vi "Athesim GUI.vi"() -> ()   [LabVIEW 2021]
uses:
  <vilib>/DAQmx/write.llb/DAQmx Write (Digital Bool 1Line 1Point).vi
  <vilib>/DAQmx/write.llb/DAQmx Write (Analog DBL 1Chan 1Samp).vi
  <vilib>/DAQmx/read.llb/DAQmx Read (Digital Bool 1Line 1Point).vi
  <vilib>/DAQmx/write.llb/DAQmx Write (Analog Wfm 1Chan NSamp).vi
  <vilib>/DAQmx/create/channels.llb/DAQmx Create Channel (DO-Digital Output).vi
  <vilib>/DAQmx/create/channels.llb/DAQmx Create Channel (DI-Digital Input).vi
  <vilib>/DAQmx/create/channels.llb/DAQmx Create Channel (AO-Voltage-Basic).vi
  <vilib>/DAQmx/miscellaneous.llb/DAQmx Fill In Error Info.vi
  <vilib>/Instr/_visa.llb/VISA Configure Serial Port (Instr).vi
  <vilib>/measure/NI_MABase.lvlib
panel:
  out "error out":errorcluster
  in  "Exposure \n(ms)":dbl=100.0
  in  "Live mode":enum32{"Static", "Strobe", "Widefield", "SIM"}(radio)=enum."Strobe"
  in  "647":bool
  in  "561":bool
  in  "488":bool
  in  "405":bool
  out "?":bool
  in  "Go live":bool
  in  "stop":bool
  in  "MG17Motor":refnum<k7>(container)
  in  "Tab Control":T1(tab)=enum."Voltages"
  in  "acquire 405":bool
  in  "405 Exp":dbl=150.0
  out "Images needed":dbl=60.0
  in  "5 phases":bool
  in  "interval /s":dbl
  in  "Timepoints":u32=5 min=1 max=1000 step=1
  in  "Steps /um":dbl
  in  "z-slices":dbl=1.0
  in  "acquire 640":bool
  in  "647 Exp":dbl=150.0
  in  "acquire 561":bool=TRUE
  in  "561 Exp":dbl=80.0
  in  "acquire 488":bool
  in  "488 Exp":dbl=150.0
  in  "Optosplit":T2(radio)=enum."rolling SIM"
  out "odd/even indicator":bool=TRUE
  out "Current voltage":dbl=0.95 format="%#_13g"
  in  "Go SIM":bool
  in  "Boolean":bool
  in  "Radio Buttons":enum32{"V1", "V2", "V3"}(radio)=enum."V3"
  in  "Debug":dbl[](array[numeric])=[0.95, 2.2, 3.45]
  out "x+y":i32=5
  in  "?":enum32{"Page 1", "Page 2", "Page 3", "Page 4"}(tab)
  in  "405 voltages":dbl[][](array[numeric])=[[1.0, 0.0, 0.0], [0.0, 0.0, 0.0], [0.0, 0.0, 4.0]]
  in  "488 voltages":dbl[][](array[numeric])=[[0.95, 2.25, 3.5], [0.951, 2.25185, 3.50055], [0.952, 2.2537, 3.5011]]
  in  "561 voltages":dbl[][](array[numeric])=[[0.95, 2.2, 3.45], [0.9506, 2.2018, 3.451], [0.9512, 2.204, 3.452]]
  in  "647 voltages":dbl[][](array[numeric])=[[0.95, 2.25, 3.5], [0.950655, 2.25185, 3.50055], [0.95131, 2.2537, 3.5011]]
  in  "?":enum32{"Page 1", "Page 2", "Page 3", "Page 4"}(tab)
  in  "405 voltages 2":dbl[][](array[numeric])=[[1.0, 0.0, 0.0], [0.0, 0.0, 0.0], [0.0, 0.0, 4.0]]
  in  "488 voltages 2":dbl[][](array[numeric])=[[0.96, 2.2, 3.5], [0.97, 2.2045, 3.51], [0.975, 2.209, 3.52]]
  in  "561 voltages 2":dbl[][](array[numeric])=[[0.85, 1.91, 3.2], [0.85065, 1.91064, 3.204], [0.85013, 1.91128, 3.208]]
  in  "647 voltages 2":dbl[][](array[numeric])=[[0.96, 2.2, 3.5], [0.97, 2.2035, 3.5085], [0.975, 2.2045, 3.5118]]
  in  "488 channel":refnum<visa-resource-name>="COM6"
  in  "ASI stage channel":refnum<visa-resource-name>="COM3"
  in  "physical channels":tag="Dev1/ao0"
  in  "expose any":tag="Dev1/port0/line5"
  in  "405 shutter":tag="Dev1/port0/line8"
  in  "Busy in":tag="Dev1/port0/line3"
  in  "Exposure out":tag="Dev1/port0/line2"
  in  "488 power":dbl(slide)=2.5974025974025974 min=0.0 max=100.0 step=0.05 scale=0.0..100.0
  in  "561 power":dbl(slide)=2.5974025974025974 min=0.0 max=100.0 step=0.05 scale=0.0..100.0
  in  "647 Power":ext(slide)=2.1 scale=0.0..100.0
  in  "488 shutter":tag="Dev1/port0/line1"
  in  "561 shutter":tag="Dev1/port0/line0"
  in  "647 channel":refnum<visa-resource-name>="COM5"
  in  "Tab Control 2":T3(tab)=enum."Page 5"
  out "Initialisation error":errorcluster
  out "stage error":errorcluster
  out "Camera/galvo error":errorcluster
  out "Laser error":errorcluster
  out "optosplit stage error":errorcluster
  out "resulting string":string="movrel z=0.000000 \r\n"
  out "resulting string 2":string="movrel z=-0.000000 \r\n"
  in  "short delay":dbl=5.0
  in  "long delay":dbl=55.0
  in  "Delay time":u32=60
  # "LIVE!"
  # "Channel"
  # "o"
  # "o"
  # "o"
  # "-60"
  # "0"
  # "60"
  # "0"
  # "2p/3"
  # "4p/3"
  # "o"
  # "o"
  # "o"
  # "-60"
  # "0"
  # "60"
  # "o"
  # "o"
  # "o"
  # "-60"
  # "0"
  # "60"
  # "o"
  # "o"
  # "o"
  # "-60"
  # "0"
  # "60"
  # "o"
  # "o"
  # "o"
  # "-60"
  # "0"
  # "60"
  # "0"
  # "3p/5"
  # "5p/5"
  # "7p/5"
  # "9p/5"
  # "o"
  # "o"
  # "o"
  # "-60"
  # "0"
  # "60"
  # "0"
  # "3p/5"
  # "5p/5"
  # "7p/5"
  # "9p/5"
  # "o"
  # "o"
  # "o"
  # "-60"
  # "0"
  # "60"
  # "0"
  # "3p/5"
  # "5p/5"
  # "7p/5"
  # "9p/5"
  # "o"
  # "o"
  # "o"
  # "-60"
  # "0"
  # "60"
  # "0"
  # "3p/5"
  # "5p/5"
  # "7p/5"
  # "9p/5"
  # "Hardware lines"
  # "Camera lines"
  # "Laser control"
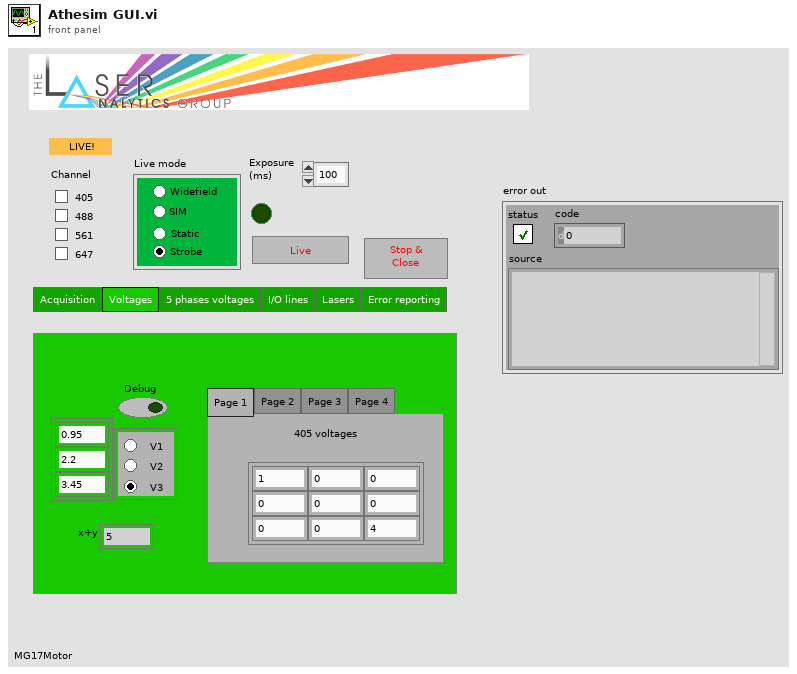
[diagram p1: front panel]
types:
  T1 = enum32{"Acquisition", "Voltages", "5 phases voltages", "I/O lines", "Lasers", "Error reporting"}
  T2 = enum32{"sequential", "optosplit", "fast sequence", "rolling SIM"}
  T3 = enum32{"Page 1", "Page 2", "Page 3", "Page 4", "Page 5"}
  T4 = enum8{"Enabled", "Disabled", "Disabled and Grayed Out"}
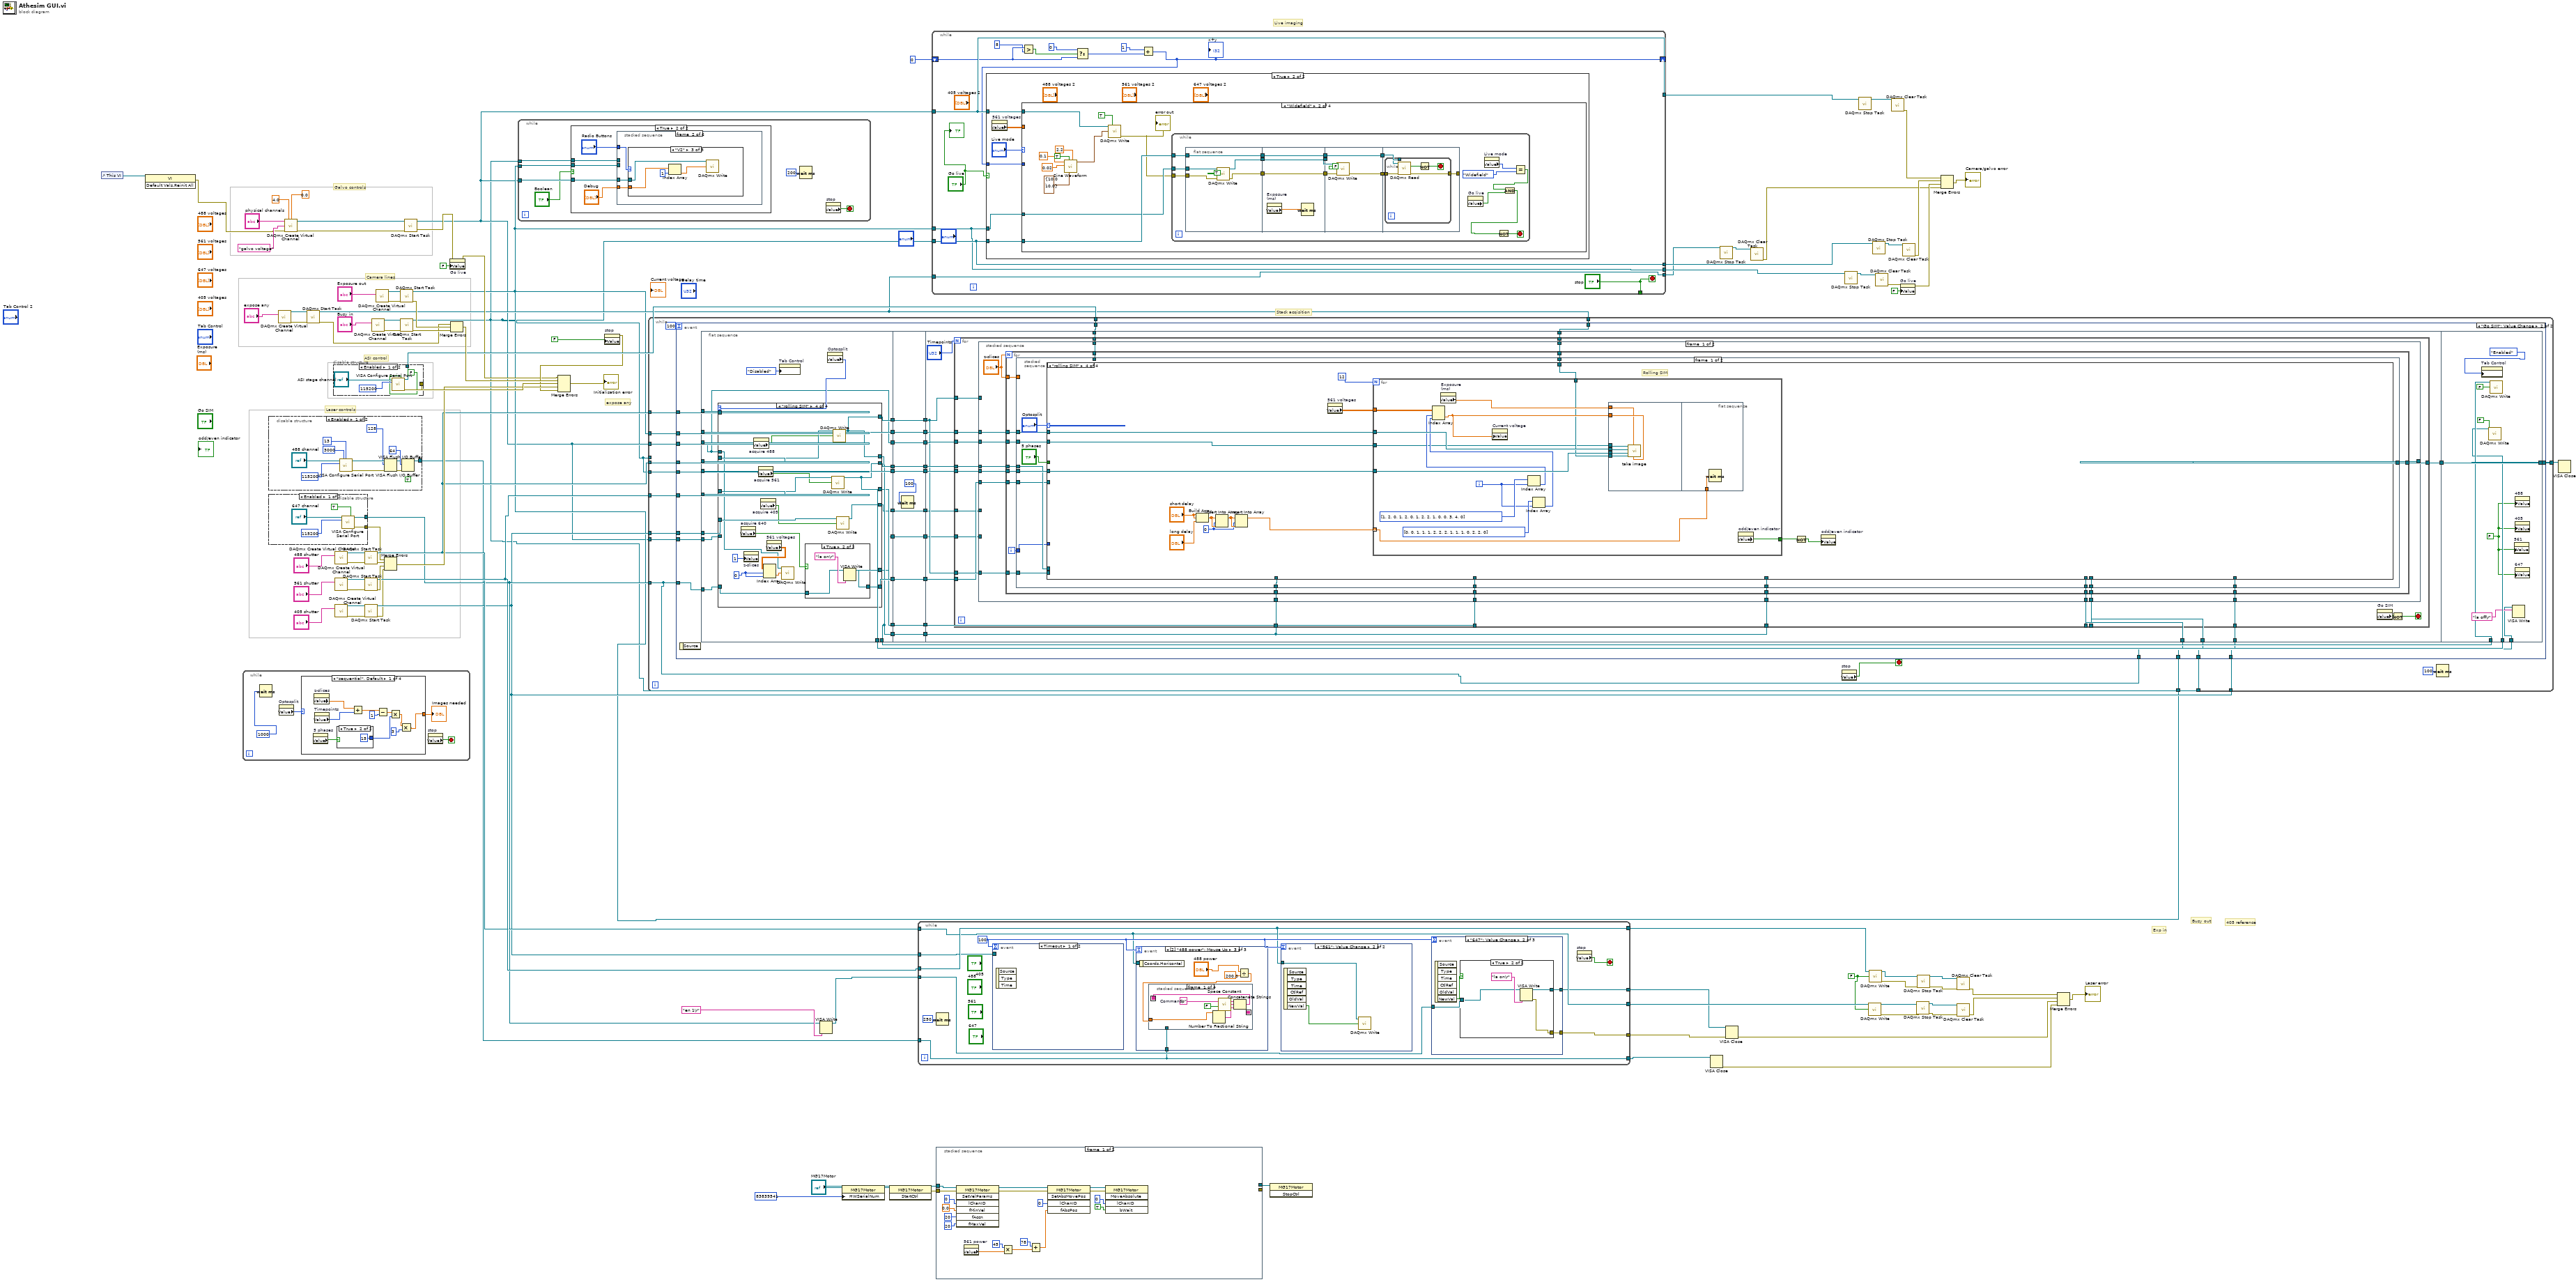
[diagram p0: block diagram]
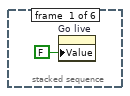
[diagram p4: hidden frame]
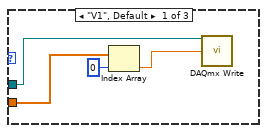
[diagram p5: hidden frame]
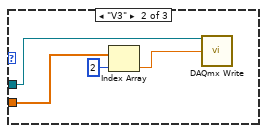
[diagram p6: hidden frame]
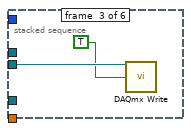
[diagram p7: hidden frame]
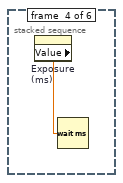
[diagram p8: hidden frame]
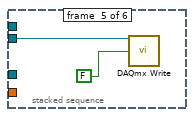
[diagram p9: hidden frame]
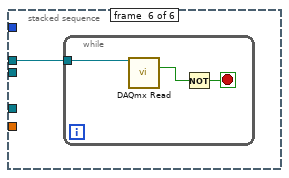
[diagram p10: hidden frame]
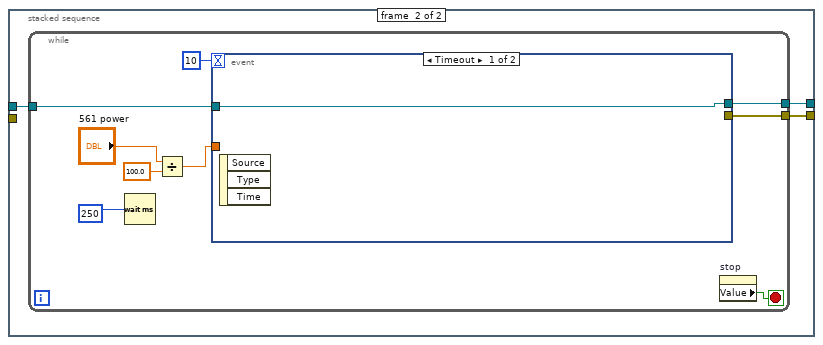
[diagram p11: hidden frame]
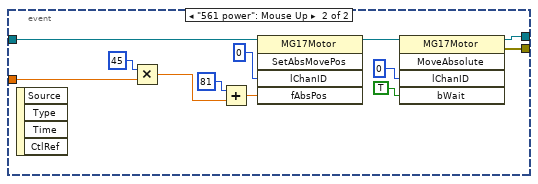
[diagram p12: hidden frame]
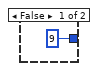
[diagram p14: hidden frame]
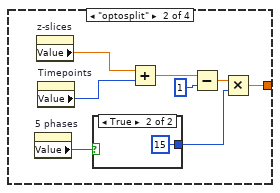
[diagram p15: hidden frame]
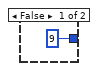
[diagram p16: hidden frame]
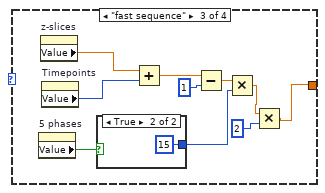
[diagram p17: hidden frame]
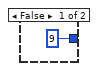
[diagram p18: hidden frame]
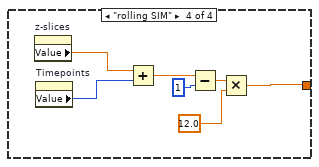
[diagram p19: hidden frame]
diagram:
  w63 = FALSE
  # "expose any"
  # "Busy out"
  # "Exp in"
  # "405 reference"
  # "Stack acqisition"
  # "Live imaging"
  # "Laser controls"
  # "ASI control"
  # "Camera lines"
  # "Galvo controls"
  n1 = control-ref of="This VI"() -> (w2:refnum<vi>)
  n2 = invoke class="VI" method="Default Vals.Reinit All"(reference=w2) -> (error out=w1:errorcluster)  [unwired: 2 in, 2 out]
  n3 = while {
    stop <- w99 stop-if-true
    n4 = Wait (ms)(milliseconds to wait=1000) -> ()  [unwired: 1 out]
    n5 = property on="Optosplit" class="RadioBtnsControl (strict)"() -> ("Value"=w98:T2)  [unwired: 2 in, 2 out]
    n6 = case shown="\"sequential\", Default" w98 {
      tunnel: [w101 w118 w123 w136] -> w100
      frame "sequential", Default {
        n7 = property on="5 phases" class="Bool (strict)"() -> ("Value"=w110:bool)  [unwired: 2 in, 2 out]
        n8 = property on="z-slices" class="DigNum (strict)"() -> ("Value"=w108:dbl)  [unwired: 2 in, 2 out]
        n9 = property on="Timepoints" class="DigNum (strict)"() -> ("Value"=w107:u32)  [unwired: 2 in, 2 out]
        n10 = case shown="True" w110 {
          tunnel: [9 15] -> w109
          frame False {
          }
          frame True {
          }
        }
        n11 = Add(x=w108, y=w107) -> (x+y=w105:dbl)
        n12 = Subtract(x=w105, y=1) -> (x-y=w104:dbl)
        n13 = Multiply(x=w104, y=w109) -> (x*y=w103:dbl)
        n14 = Multiply(x=w103, y=3) -> (x*y=w101:dbl)
      }
      frame "optosplit" {
        n15 = property on="5 phases" class="Bool (strict)"() -> ("Value"=w120:bool)  [unwired: 2 in, 2 out]
        n16 = property on="z-slices" class="DigNum (strict)"() -> ("Value"=w117:dbl)  [unwired: 2 in, 2 out]
        n17 = property on="Timepoints" class="DigNum (strict)"() -> ("Value"=w116:u32)  [unwired: 2 in, 2 out]
        n18 = case shown="True" w120 {
          tunnel: [9 15] -> w119
          frame False {
          }
          frame True {
          }
        }
        n19 = Add(x=w117, y=w116) -> (x+y=w114:dbl)
        n20 = Subtract(x=w114, y=1) -> (x-y=w113:dbl)
        n21 = Multiply(x=w113, y=w119) -> (x*y=w118:dbl)
      }
      frame "fast sequence" {
        n22 = property on="5 phases" class="Bool (strict)"() -> ("Value"=w132:bool)  [unwired: 2 in, 2 out]
        n23 = property on="z-slices" class="DigNum (strict)"() -> ("Value"=w130:dbl)  [unwired: 2 in, 2 out]
        n24 = property on="Timepoints" class="DigNum (strict)"() -> ("Value"=w129:u32)  [unwired: 2 in, 2 out]
        n25 = case shown="True" w132 {
          tunnel: [9 15] -> w131
          frame False {
          }
          frame True {
          }
        }
        n26 = Add(x=w130, y=w129) -> (x+y=w127:dbl)
        n27 = Subtract(x=w127, y=1) -> (x-y=w126:dbl)
        n28 = Multiply(x=w126, y=w131) -> (x*y=w125:dbl)
        n29 = Multiply(x=w125, y=2) -> (x*y=w123:dbl)
      }
      frame "rolling SIM" {
        n30 = property on="z-slices" class="DigNum (strict)"() -> ("Value"=w141:dbl)  [unwired: 2 in, 2 out]
        n31 = property on="Timepoints" class="DigNum (strict)"() -> ("Value"=w140:u32)  [unwired: 2 in, 2 out]
        n32 = Add(x=w141, y=w140) -> (x+y=w138:dbl)
        n33 = Subtract(x=w138, y=1) -> (x-y=w137:dbl)
        n34 = Multiply(x=w137, y=12.0) -> (x*y=w136:dbl)
      }
    }
    "Images needed" <- w100
    n35 = property on="stop" class="Bool (strict)"() -> ("Value"=w99:bool)  [unwired: 2 in, 2 out]
  }
  n36 = disable-structure shown="Enabled" {
    disable-tunnel: [w142 _] -> w6
    frame Enabled {
      (unwired) TRUE ("Enable Termination\nChar (T)")
      n37 = call-poly "VISA Configure Serial Port"("VISA resource name"="488 channel", "timeout (10sec)"=u32 3000, "termination char\n(0xA = '\\n' = LF)"=u8 13 ("termination char\n(0xA = '\\n' = LF)"), "baud rate (9600)"=u32 115200) -> ("VISA resource name out"=w152:refnum<visa-resource-name>, "error out"=w151:errorcluster)  [unwired: 5 in, 5 out]
      n38 = VISA Flush I/O Buffer(VISA resource name=w152, mask (16)=u16 128, error in (no error)=w151) -> (VISA resource name out=w148:refnum<visa-resource-name>, error out=w147:errorcluster)
      n39 = VISA Flush I/O Buffer(VISA resource name=w148, mask (16)=u16 64, error in (no error)=w147) -> (VISA resource name out=w142:refnum<visa-resource-name>)  [unwired: 1 out]
    }
    frame Disabled {
    }
  }
  n40 = disable-structure shown="Enabled" {
    disable-tunnel: [w154 _] -> w33
    disable-tunnel: [w153 _] -> w35
    frame Enabled {
      n41 = call-poly "VISA Configure Serial Port"("VISA resource name"="647 channel", "Enable Termination\nChar (T)"=TRUE ("Enable Termination\nChar (T)"), "baud rate (9600)"=u32 115200) -> ("VISA resource name out"=w154:refnum<visa-resource-name>, "error out"=w153:errorcluster)  [unwired: 11 in]
    }
    frame Disabled {
    }
  }
  n42 = call-poly <vilib>:"DAQmx Create Virtual Channel.vi"("lines"="expose any") -> ("task out"=w19:refnum<k21>, "error out"=w18:errorcluster)  [unwired: 13 in]
  n43 = call-poly <vilib>:"DAQmx Create Virtual Channel.vi"("maximum value"=4.0, "minimum value"=0.0, "physical channels"="physical channels", "name to assign"="galvo voltage", "error in"=w1) -> ("task out"=w12:refnum<k21>, "error out"=w11:errorcluster)  [unwired: 9 in]
  n44 = call <vilib>:"DAQmx Start Task.vi"("task/channels in"=w19, "error in"=w18) -> ("task out"=w16:refnum<k21>, "error out"=w17:errorcluster)  [unwired: 12 in]
  n45 = disable-structure shown="Enabled" {
    disable-tunnel: [w160 _] -> w80
    disable-tunnel: [w159 _] -> w51
    frame Enabled {
      n46 = call-poly "VISA Configure Serial Port"("VISA resource name"="ASI stage channel", "Enable Termination\nChar (T)"=FALSE, "baud rate (9600)"=u32 115200) -> ("VISA resource name out"=w159:refnum<visa-resource-name>, "error out"=w160:errorcluster)  [unwired: 11 in]
    }
    frame Disabled {
    }
  }
  n47 = call-poly <vilib>:"DAQmx Create Virtual Channel.vi"("lines"="488 shutter") -> ("task out"=w91:refnum<k21>, "error out"=w92:errorcluster)  [unwired: 13 in]
  n48 = call-poly <vilib>:"DAQmx Create Virtual Channel.vi"("lines"="561 shutter") -> ("task out"=w89:refnum<k21>, "error out"=w90:errorcluster)  [unwired: 13 in]
  n49 = call-poly <vilib>:"DAQmx Create Virtual Channel.vi"("lines"="405 shutter") -> ("task out"=w45:refnum<k21>, "error out"=w46:errorcluster)  [unwired: 13 in]
  n50 = call <vilib>:"DAQmx Start Task.vi"("task/channels in"=w91, "error in"=w92) -> ("task out"=w75:refnum<k21>, "error out"=w84:errorcluster)  [unwired: 12 in]
  n51 = call <vilib>:"DAQmx Start Task.vi"("task/channels in"=w89, "error in"=w90) -> ("task out"=w76:refnum<k21>, "error out"=w83:errorcluster)  [unwired: 12 in]
  n52 = call <vilib>:"DAQmx Start Task.vi"("task/channels in"=w45, "error in"=w46) -> ("task out"=w31:refnum<k21>, "error out"=w7:errorcluster)  [unwired: 12 in]
  n53 = call-poly <vilib>:"DAQmx Create Virtual Channel.vi"("lines"="Busy in") -> ("task out"=w93:refnum<k21>, "error out"=w94:errorcluster)  [unwired: 13 in]
  n54 = call-poly <vilib>:"DAQmx Create Virtual Channel.vi"("lines"="Exposure out") -> ("task out"=w96:refnum<k21>, "error out"=w95:errorcluster)  [unwired: 13 in]
  n55 = Merge Errors(w35, w84, w83, w7) -> (w78:errorcluster)
  n56 = call <vilib>:"DAQmx Start Task.vi"("task/channels in"=w96, "error in"=w95) -> ("task out"=w9:refnum<k21>, "error out"=w82:errorcluster)  [unwired: 12 in]
  n57 = call <vilib>:"DAQmx Start Task.vi"("task/channels in"=w93, "error in"=w94) -> ("task out"=w3:refnum<k21>, "error out"=w81:errorcluster)  [unwired: 12 in]
  n58 = call <vilib>:"DAQmx Start Task.vi"("task/channels in"=w12, "error in"=w11) -> ("task out"=w8:refnum<k21>, "error out"=w29:errorcluster)  [unwired: 12 in]
  n59 = property on="Go live" class="Bool (strict)"(error in=w29, "Value"=FALSE) -> (error out=w28:errorcluster)  [unwired: 1 in, 1 out]
  n60 = Merge Errors(w17, w82, w81) -> (w79:errorcluster)
  n61 = while {
    tunnel: w9 -> [w167]
    tunnel: w3 -> [w166]
    tunnel: w8 -> [w165]
    stop <- w168 stop-if-true
    n62 = case shown="True" "Boolean" {
      tunnel: w167 -> [_ w173]
      tunnel: w166 -> [_ w172]
      tunnel: w165 -> [_ w171]
      frame False {
      }
      frame True {
        n63 = stacked-sequence {
          tunnel: w173 -> [_ _ w191 _ w193 _]
          tunnel: w172 -> [_ _ _ _ _ w195]
          tunnel: "Radio Buttons" -> [_ w177 _ _ _ _]
          tunnel: "Debug" -> [_ w176 _ _ _ _]
          tunnel: w171 -> [_ w175 _ _ _ _]
          frame #0 {
            n64 = property on="Go live" class="Bool (strict)"("Value"=FALSE ("Go live")) -> ()  [unwired: 2 in, 2 out]
          }
          frame #1 {
            n65 = case shown="\"V2\"" w177 {
              tunnel: w176 -> [w180 w184 w188]
              tunnel: w175 -> [w181 w185 w189]
              frame "V1", Default {
                n66 = Index Array(array=w180, index=0) -> (element=w179:dbl)
                n67 = call-poly <vilib>:"DAQmx Write.vi"("task/channels in"=w181, "data"=w179) -> ()  [unwired: 11 in, 3 out]
              }
              frame "V3" {
                n68 = Index Array(array=w184, index=2) -> (element=w183:dbl)
                n69 = call-poly <vilib>:"DAQmx Write.vi"("task/channels in"=w185, "data"=w183) -> ()  [unwired: 11 in, 3 out]
              }
              frame "V2" {
                n70 = Index Array(array=w188, index=1) -> (element=w187:dbl)
                n71 = call-poly <vilib>:"DAQmx Write.vi"("task/channels in"=w189, "data"=w187) -> ()  [unwired: 11 in, 3 out]
              }
            }
          }
          frame #2 {
            n72 = call-poly <vilib>:"DAQmx Write.vi"("task/channels in"=w191, "data"=TRUE) -> ()  [unwired: 11 in, 3 out]
          }
          frame #3 {
            n73 = property on="Exposure \n(ms)" class="DigNum (strict)"() -> ("Value"=w192:dbl)  [unwired: 2 in, 2 out]
            n74 = Wait (ms)(milliseconds to wait=w192) -> ()  [unwired: 1 out]
          }
          frame #4 {
            n75 = call-poly <vilib>:"DAQmx Write.vi"("task/channels in"=w193, "data"=FALSE) -> ()  [unwired: 11 in, 3 out]
          }
          frame #5 {
            n76 = while {
              tunnel: w195 -> [w196]
              stop <- w198 stop-if-true
              n77 = call-poly <vilib>:"DAQmx Read.vi"("task/channels in"=w196) -> ("data"=w197:bool)  [unwired: 12 in, 2 out]
              n78 = Not(x=w197) -> (.not. x?=w198:bool)
            }
          }
        }
      }
    }
    n79 = Wait (ms)(milliseconds to wait=u32 200) -> ()  [unwired: 1 out]
    n80 = property on="stop" class="Bool (strict)"() -> ("Value"=w168:bool)  [unwired: 2 in, 2 out]
  }
  n81 = property on="stop" class="Bool (strict)"("Value"=FALSE) -> (error out=w48:errorcluster)  [unwired: 2 in, 1 out]
  n82 = Merge Errors(w28, w79, w80, w78, w48) -> (→"Initialisation error":errorcluster)
  n83 = while {
    tunnel: w9 -> [w215]
    tunnel: w3 -> [w214]
    tunnel: w8 -> [w213]
    tunnel: w75 -> [w212]
    tunnel: w76 -> [w211]
    tunnel: w75 -> [w210]
    tunnel: w51 -> [w208]
    tunnel: [w207] -> w50
    tunnel: w3 -> [_]
    tunnel: w33 -> [w205]
    tunnel: w31 -> [w206]
    tunnel: w31 -> [w204]
    tunnel: w9 -> [w203]
    tunnel: w3 -> [w202]
    tunnel: w8 -> [w201]
    tunnel: w16 -> [w200]
    stop <- w209 stop-if-true
    n84 = event shown="[1] \"Go SIM\": Value Change" {
      selector: _ -> [_ _]
      dyn-events: _ -> [_ _]
      timeout: 100 -> [_ _]
      tunnel: w215 -> [_ w256]
      tunnel: w214 -> [_ w255]
      tunnel: w213 -> [_ w254]
      tunnel: w212 -> [_ w253]
      tunnel: w211 -> [_ w252]
      tunnel: w210 -> [_ w251]
      tunnel: w208 -> [w217 w250]
      tunnel: [w217 w249] -> w207
      tunnel: w205 -> [_ w245]
      tunnel: w206 -> [_ w244]
      tunnel: w205 -> [_ w243]
      tunnel: w204 -> [_ w242]
      tunnel: w203 -> [_ w241]
      tunnel: w202 -> [_ w240]
      tunnel: w201 -> [_ w239]
      tunnel: w200 -> [_ w218]
      event Timeout {
        n85 = event-data() -> ()  [unwired: 1 in, 3 out]
      }
      event "Go SIM": Value Change {
        n86 = event-data() -> ()  [unwired: 1 in, 1 out]
        n87 = flat-sequence {
          tunnel: [w274] -> w238
          tunnel: w256 -> [w274]
          tunnel: [w273] -> w236
          tunnel: w255 -> [w273]
          tunnel: [w258] -> w234
          tunnel: w254 -> [w258]
          tunnel: w253 -> [w271]
          tunnel: w252 -> [w270]
          tunnel: w251 -> [w269]
          tunnel: [w268] -> w232
          tunnel: [w267] -> w230
          tunnel: [w263] -> w246
          tunnel: [w262] -> w247
          tunnel: w245 -> [w266]
          tunnel: w244 -> [w265]
          tunnel: [w264] -> w228
          tunnel: [w263] -> w226
          tunnel: [w262] -> w224
          tunnel: w239 -> [w261]
          tunnel: [w260] -> w221
          tunnel: [w259] -> w219
          tunnel: w238 -> [w364]
          tunnel: [w364] -> w237
          tunnel: w236 -> [w363]
          tunnel: [w363] -> w235
          tunnel: w234 -> [w362]
          tunnel: [w362] -> w233
          tunnel: w232 -> [w361]
          tunnel: [w361] -> w231
          tunnel: w230 -> [w360]
          tunnel: [w360] -> w229
          tunnel: w228 -> [w359]
          tunnel: [w359] -> w227
          tunnel: w226 -> [w358]
          tunnel: [w358] -> w225
          tunnel: w224 -> [w357]
          tunnel: [w357] -> w223
          tunnel: [w355] -> w222
          tunnel: w221 -> [w355]
          tunnel: [w354] -> w220
          tunnel: w219 -> [w354]
          tunnel: w237 -> [w381]
          tunnel: w235 -> [w380]
          tunnel: w233 -> [w379]
          tunnel: w231 -> [w378]
          tunnel: w229 -> [w369]
          tunnel: w250 -> [w377]
          tunnel: [w376] -> w248
          tunnel: w227 -> [w375]
          tunnel: w225 -> [w373]
          tunnel: w223 -> [w374]
          tunnel: w242 -> [w372]
          tunnel: w241 -> [w371]
          tunnel: w240 -> [w370]
          tunnel: w222 -> [w368]
          tunnel: w220 -> [w367]
          tunnel: w218 -> [w366]
          tunnel: [w1176] -> w249
          tunnel: w248 -> [w1176]
          tunnel: w247 -> [w1172]
          tunnel: w246 -> [w1173]
          tunnel: w243 -> [w1170]
          frame #0 {
            n88 = property on="Tab Control" class="TabCtl (strict)"("DisabledEnum"=T4."Disabled" ("Disabled")) -> ()  [unwired: 2 in, 2 out]
            n89 = property on="Optosplit" class="RadioBtnsControl (strict)"() -> ("Value"=w272:T2)  [unwired: 2 in, 2 out]
            n90 = case shown="\"rolling SIM\"" w272 {
              tunnel: w271 -> [_ _ _ _]
              tunnel: w270 -> [w285 w307 w326 w345]
              tunnel: w269 -> [w286 w308 w328 w347]
              tunnel: [w284 w306 w325 w344] -> w268
              tunnel: [w283 w305 w327 w346] -> w267
              tunnel: [w284 w306 w325 w344] -> w262
              tunnel: [w283 w305 w327 w346] -> w263
              tunnel: w266 -> [w278 w300 w323 w343]
              tunnel: w265 -> [w281 w303 w321 w342]
              tunnel: [w275 w297 w319 w340] -> w264
              tunnel: [w279 w301 w320 w341] -> w260
              tunnel: w261 -> [w276 w299 _ _]
              tunnel: [w275 w297 w319 w340] -> w259
              tunnel: w258 -> [_ _ _ w331]
              frame "sequential", Default {
                n91 = property on="odd/even indicator" class="Bool (strict)"() -> ("Value"=w277:bool)  [unwired: 2 in, 2 out]
                n92 = case shown="True" w277 {
                  tunnel: w276 -> [w292 w296]
                  frame False {
                    w290 = 2
                    n93 = property on="647 voltages" class="Arr (strict)"() -> ("Value"=w291:dbl[][])  [unwired: 2 in, 2 out]
                    n94 = Index Array(array=w291, index (row)=w290, index (col)=w290) -> (element=w289:dbl)
                    n95 = call-poly <vilib>:"DAQmx Write.vi"("task/channels in"=w292, "data"=w289) -> ()  [unwired: 11 in, 3 out]
                  }
                  frame True {
                    w294 = 0
                    n96 = property on="561 voltages" class="Arr (strict)"() -> ("Value"=w295:dbl[][])  [unwired: 2 in, 2 out]
                    n97 = Index Array(array=w295, index (row)=w294, index (col)=w294) -> (element=w293:dbl)
                    n98 = call-poly <vilib>:"DAQmx Write.vi"("task/channels in"=w296, "data"=w293) -> ()  [unwired: 11 in, 3 out]
                  }
                }
                n99 = call-poly <vilib>:"DAQmx Write.vi"("task/channels in"=w281, "data"=FALSE) -> ("task out"=w279:refnum<k21>)  [unwired: 11 in, 2 out]
                n100 = call-poly <vilib>:"DAQmx Write.vi"("task/channels in"=w285, "data"=FALSE) -> ("task out"=w284:refnum<k21>)  [unwired: 11 in, 2 out]
                n101 = call-poly <vilib>:"DAQmx Write.vi"("task/channels in"=w286, "data"=FALSE) -> ("task out"=w283:refnum<k21>)  [unwired: 11 in, 2 out]
                n102 = VISA Write(VISA resource name=w278, write buffer="la off\r" ("format string")) -> (VISA resource name out=w275:refnum<visa-resource-name>)  [unwired: 1 in, 2 out]
              }
              frame "fast sequence" {
                n103 = property on="odd/even indicator" class="Bool (strict)"() -> ("Value"=w298:bool)  [unwired: 2 in, 2 out]
                n104 = case shown="True" w298 {
                  tunnel: w299 -> [w314 w318]
                  frame False {
                    w312 = 2
                    n105 = property on="647 voltages" class="Arr (strict)"() -> ("Value"=w313:dbl[][])  [unwired: 2 in, 2 out]
                    n106 = Index Array(array=w313, index (row)=w312, index (col)=w312) -> (element=w311:dbl)
                    n107 = call-poly <vilib>:"DAQmx Write.vi"("task/channels in"=w314, "data"=w311) -> ()  [unwired: 11 in, 3 out]
                  }
                  frame True {
                    w316 = 0
                    n108 = property on="647 voltages" class="Arr (strict)"() -> ("Value"=w317:dbl[][])  [unwired: 2 in, 2 out]
                    n109 = Index Array(array=w317, index (row)=w316, index (col)=w316) -> (element=w315:dbl)
                    n110 = call-poly <vilib>:"DAQmx Write.vi"("task/channels in"=w318, "data"=w315) -> ()  [unwired: 11 in, 3 out]
                  }
                }
                n111 = call-poly <vilib>:"DAQmx Write.vi"("task/channels in"=w303, "data"=FALSE) -> ("task out"=w301:refnum<k21>)  [unwired: 11 in, 2 out]
                n112 = call-poly <vilib>:"DAQmx Write.vi"("task/channels in"=w307, "data"=FALSE) -> ("task out"=w306:refnum<k21>)  [unwired: 11 in, 2 out]
                n113 = call-poly <vilib>:"DAQmx Write.vi"("task/channels in"=w308, "data"=FALSE) -> ("task out"=w305:refnum<k21>)  [unwired: 11 in, 2 out]
                n114 = VISA Write(VISA resource name=w300, write buffer="la off\r" ("format string")) -> (VISA resource name out=w297:refnum<visa-resource-name>)  [unwired: 1 in, 2 out]
              }
              frame "optosplit" {
                n115 = call-poly <vilib>:"DAQmx Write.vi"("task/channels in"=w326, "data"=TRUE) -> ("task out"=w325:refnum<k21>)  [unwired: 11 in, 2 out]
                n116 = call-poly <vilib>:"DAQmx Write.vi"("task/channels in"=w328, "data"=TRUE) -> ("task out"=w327:refnum<k21>)  [unwired: 11 in, 2 out]
                n117 = call-poly <vilib>:"DAQmx Write.vi"("task/channels in"=w321, "data"=TRUE) -> ("task out"=w320:refnum<k21>)  [unwired: 11 in, 2 out]
                n118 = VISA Write(VISA resource name=w323, write buffer="la on\r" ("format string")) -> (VISA resource name out=w319:refnum<visa-resource-name>)  [unwired: 1 in, 2 out]
              }
              frame "rolling SIM" {
                w336 = 0
                n119 = property on="acquire 640" class="Bool (strict)"() -> ("Value"=w332:bool)  [unwired: 2 in, 2 out]
                n120 = property on="z-slices" class="DigNum (strict)"("Value"=1) -> ()  [unwired: 2 in, 2 out]
                n121 = property on="acquire 488" class="Bool (strict)"() -> ("Value"=w335:bool)  [unwired: 2 in, 2 out]
                n122 = property on="acquire 561" class="Bool (strict)"() -> ("Value"=w334:bool)  [unwired: 2 in, 2 out]
                n123 = property on="acquire 405" class="Bool (strict)"() -> ("Value"=w333:bool)  [unwired: 2 in, 2 out]
                n124 = property on="561 voltages" class="Arr (strict)"() -> ("Value"=w337:dbl[][])  [unwired: 2 in, 2 out]
                n125 = Index Array(array=w337, index (row)=w336, index (col)=w336) -> (element=w338:dbl)
                n126 = call-poly <vilib>:"DAQmx Write.vi"("task/channels in"=w331, "data"=w338) -> ()  [unwired: 11 in, 3 out]
                n127 = case shown="True" w332 {
                  tunnel: w343 -> [w349 w352]
                  tunnel: [w348 w351] -> w340
                  frame False {
                    n128 = VISA Write(VISA resource name=w349, write buffer="la off\r" ("format string")) -> (VISA resource name out=w348:refnum<visa-resource-name>)  [unwired: 1 in, 2 out]
                  }
                  frame True {
                    n129 = VISA Write(VISA resource name=w352, write buffer="la on\r" ("format string")) -> (VISA resource name out=w351:refnum<visa-resource-name>)  [unwired: 1 in, 2 out]
                  }
                }
                n130 = call-poly <vilib>:"DAQmx Write.vi"("task/channels in"=w345, "data"=w334) -> ("task out"=w344:refnum<k21>)  [unwired: 11 in, 2 out]
                n131 = call-poly <vilib>:"DAQmx Write.vi"("task/channels in"=w347, "data"=w335) -> ("task out"=w346:refnum<k21>)  [unwired: 11 in, 2 out]
                n132 = call-poly <vilib>:"DAQmx Write.vi"("task/channels in"=w342, "data"=w333) -> ("task out"=w341:refnum<k21>)  [unwired: 11 in, 2 out]
              }
            }
          }
          frame #1 {
            n133 = Wait (ms)(milliseconds to wait=100) -> ()  [unwired: 1 out]
          }
          frame #2 {
            n134 = for {
              N: "Timepoints" -> [_]
              tunnel: w381 -> [w401]
              tunnel: w380 -> [w400]
              tunnel: w379 -> [w399]
              tunnel: w378 -> [w398]
              tunnel: w369 -> [w397]
              tunnel: w377 -> [w396]
              tunnel: [w395] -> w376
              tunnel: w375 -> [w394]
              tunnel: w374 -> [w393]
              tunnel: w373 -> [w392]
              tunnel: w373 -> [w391]
              tunnel: w372 -> [w390]
              tunnel: w371 -> [w389]
              tunnel: w370 -> [w388]
              tunnel: w369 -> [w387]
              tunnel: w368 -> [w386]
              tunnel: w367 -> [w385]
              tunnel: w366 -> [w384]
              stop <- w382 stop-if-true
              n135 = stacked-sequence {
                tunnel: w401 -> [w417 _]
                tunnel: w400 -> [w416 _]
                tunnel: w399 -> [w415 _]
                tunnel: w398 -> [w414 w1081]
                tunnel: w397 -> [w413 _]
                tunnel: w396 -> [w412 w1083]
                tunnel: [w411 _] -> w395
                tunnel: w394 -> [w410 _]
                tunnel: w393 -> [w409 _]
                tunnel: w392 -> [w408 _]
                tunnel: w391 -> [w407 _]
                tunnel: w390 -> [w406 _]
                tunnel: w389 -> [w405 _]
                tunnel: w388 -> [w404 _]
                tunnel: w387 -> [_ w1082]
                tunnel: w386 -> [_ w1080]
                tunnel: w385 -> [_ w1079]
                tunnel: w384 -> [w402 _]
                frame #0 {
                  n136 = for {
                    N: "z-slices" -> [_]
                    tunnel: w417 -> [w434]
                    tunnel: w416 -> [w433]
                    tunnel: w415 -> [w432]
                    tunnel: w414 -> [w431]
                    tunnel: w413 -> [w430]
                    tunnel: w412 -> [w429]
                    tunnel: [w428] -> w411
                    tunnel: w410 -> [w427]
                    tunnel: w409 -> [w426]
                    tunnel: w408 -> [w425]
                    tunnel: w407 -> [w424]
                    tunnel: w406 -> [w423]
                    tunnel: w405 -> [w422]
                    tunnel: w404 -> [w421]
                    tunnel: "z-slices" -> [w419]
                    tunnel: w402 -> [w418]
                    i -> [w420]
                    n137 = stacked-sequence {
                      tunnel: w434 -> [w449 _]
                      tunnel: w433 -> [w448 _]
                      tunnel: w432 -> [w447 _]
                      tunnel: w431 -> [w446 _]
                      tunnel: w430 -> [w445 _]
                      tunnel: w429 -> [_ w1051]
                      tunnel: [_ w1050] -> w428
                      tunnel: w427 -> [w443 _]
                      tunnel: w426 -> [w442 _]
                      tunnel: w425 -> [w441 _]
                      tunnel: w424 -> [w440 _]
                      tunnel: w423 -> [w439 _]
                      tunnel: w422 -> [w438 _]
                      tunnel: w421 -> [w437 _]
                      tunnel: w420 -> [w436 _]
                      tunnel: w419 -> [_ w1046]
                      tunnel: w418 -> [w435 _]
                      frame #0 {
                        n138 = case shown="\"rolling SIM\"" "Optosplit" {
                          tunnel: w449 -> [w472 w795 w924 w1021]
                          tunnel: w448 -> [w471 w794 w923 w1020]
                          tunnel: w447 -> [w454 w790 w922 w1014]
                          tunnel: w446 -> [w461 _ _ _]
                          tunnel: w445 -> [w460 _ _ _]
                          tunnel: "5 phases" -> [_ _ w921 _]
                          tunnel: w443 -> [w459 w789 _ _]
                          tunnel: w442 -> [w458 w788 _ _]
                          tunnel: w441 -> [w457 _ _ _]
                          tunnel: w440 -> [_ w783 _ _]
                          tunnel: w439 -> [w456 w782 _ _]
                          tunnel: w438 -> [w453 _ _ _]
                          tunnel: w437 -> [w452 _ _ _]
                          tunnel: w436 -> [_ _ _ _]
                          tunnel: w435 -> [w451 w781 w920 w1015]
                          frame "sequential", Default {
                            # "Without optosplit"
                            n139 = case shown="True" "acquire 640" {
                              tunnel: w472 -> [w700 w710]
                              tunnel: w471 -> [w698 w709]
                              tunnel: w454 -> [w699 w703]
                              tunnel: [w700 w707] -> w467
                              tunnel: [w699 w708] -> w468
                              tunnel: [w698 w706] -> w469
                              tunnel: w459 -> [_ w702]
                              tunnel: w451 -> [_ w701]
                              frame False {
                              }
                              frame True {
                                n140 = property on="647 voltages" class="Arr (strict)"() -> ("Value"=w704:dbl[][])  [unwired: 2 in, 2 out]
                                n141 = stacked-sequence {
                                seq-local: [_ w724 _ _] -> [_ _ w744 _]
                                seq-local: [_ w723 _ _] -> [_ _ w743 _]
                                seq-local: [_ w722 _ _] -> [_ _ w742 _]
                                seq-local: [_ w721 _ _] -> [_ _ w738 _]
                                seq-local: [_ w720 _ _] -> [_ _ w737 _]
                                tunnel: w710 -> [_ w724 _ _]
                                tunnel: w703 -> [_ w723 _ _]
                                tunnel: w709 -> [_ w722 _ _]
                                tunnel: w704 -> [_ w721 _ _]
                                tunnel: "647 Exp" -> [_ w720 _ _]
                                tunnel: [_ _ w741 _] -> w708
                                tunnel: [_ _ w740 _] -> w707
                                tunnel: [_ _ w739 _] -> w706
                                tunnel: w704 -> [_ w719 _ _]
                                tunnel: w703 -> [_ w718 _ _]
                                tunnel: w702 -> [w711 _ _ w778]
                                tunnel: w701 -> [_ _ w735 _]
                                frame #0 {
                                n142 = stacked-sequence {
                                tunnel: w711 -> [w712 _]
                                frame #0 {
                                n143 = VISA Write(VISA resource name=w712, write buffer="la on\r" ("format string")) -> ()  [unwired: 1 in, 3 out]
                                }
                                frame #1 {
                                n144 = Wait (ms)(milliseconds to wait=100) -> ()  [unwired: 1 out]
                                }
                                }
                                }
                                frame #1 {
                                n145 = property on="odd/even indicator" class="Bool (strict)"() -> ("Value"=w715:bool)  [unwired: 2 in, 2 out]
                                n146 = case shown="False" w715 {
                                tunnel: [2 0] -> w717
                                tunnel: [2 0] -> w716
                                frame False {
                                }
                                frame True {
                                }
                                }
                                n147 = flat-sequence {
                                tunnel: [w732] -> _
                                tunnel: w719 -> [w734]
                                tunnel: w718 -> [w732]
                                tunnel: [w733] -> _
                                tunnel: w717 -> [w730]
                                tunnel: w716 -> [w729]
                                frame #0 {
                                n148 = Index Array(array=w734, index (row)=w730, index (col)=w729) -> (element=w731:dbl)
                                n149 = call-poly <vilib>:"DAQmx Write.vi"("task/channels in"=w732, "data"=w731) -> ("task out"=w733:refnum<k21>)  [unwired: 11 in, 2 out]
                                }
                                }
                                }
                                frame #2 {
                                n150 = for {
                                N: 9 -> [_]
                                tunnel: w738 -> [w756]
                                tunnel: w744 -> [w753]
                                tunnel: w743 -> [w754]
                                tunnel: w742 -> [w752]
                                tunnel: w737 -> [w755]
                                tunnel: [w754] -> w741
                                tunnel: [w753] -> w740
                                tunnel: [w752] -> w739
                                tunnel: w735 -> [w745]
                                i -> [w748]
                                n151 = property on="odd/even indicator" class="Bool (strict)"() -> ("Value"=w746:bool)  [unwired: 2 in, 2 out]
                                n152 = case shown="True" w746 {
                                tunnel: [i32[] [1, 0, 2, 1, 0, 2, 1, 0, 0, 0, 1, 2, 3, 4, 0] i32[] [1, 2, 0, 1, 2, 0, 1, 2, 2, 0, 1, 2, 3, 4, 0]] -> w751
                                tunnel: [i32[] [2, 2, 1, 1, 1, 0, 0, 0, 0, 2, 2, 2, 2, 2, 0] i32[] [0, 0, 1, 1, 1, 2, 2, 2, 2, 2, 2, 2, 2, 2, 0]] -> w750
                                frame False {
                                }
                                frame True {
                                }
                                }
                                n153 = Index Array(array=w751, index=w748) -> (element=w749:i32)
                                n154 = flat-sequence {
                                tunnel: w756 -> [w765]
                                tunnel: w755 -> [w769]
                                tunnel: w754 -> [w768]
                                tunnel: w753 -> [w767]
                                tunnel: w752 -> [w766]
                                tunnel: w747 -> [w763]
                                tunnel: w749 -> [w762]
                                tunnel: w745 -> [w761]
                                frame #0 {
                                n155 = Index Array(array=w765, index (row)=w762, index (col)=w763) -> (element=w764:dbl)
                                n156 = call "take image.vi"("Voltage"=w764, "Exposure time"=w769, "expose any"=w761, "Busy out"=w766, "Exp In"=w767, "Galvo"=w768) -> ()  [unwired: 6 in]
                                }
                                frame #1 {
                                n157 = property on="Delay time" class="DigNum (strict)"() -> ("Value"=w770:u32)  [unwired: 2 in, 2 out]
                                n158 = Wait (ms)(milliseconds to wait=w770) -> ()  [unwired: 1 out]
                                }
                                }
                                n159 = Index Array(array=w750, index=w748) -> (element=w747:i32)
                                }
                                }
                                frame #3 {
                                n160 = property on="acquire 488" class="Bool (strict)"() -> ("Value"=w774:bool)  [unwired: 2 in, 2 out]
                                n161 = property on="acquire 405" class="Bool (strict)"() -> ("Value"=w773:bool)  [unwired: 2 in, 2 out]
                                n162 = property on="acquire 561" class="Bool (strict)"() -> ("Value"=w775:bool)  [unwired: 2 in, 2 out]
                                n163 = property on="odd/even indicator" class="Bool (strict)"() -> ("Value"=w776:bool)  [unwired: 2 in, 2 out]
                                n164 = Or(x=w775, y=w774) -> (x .or. y?=w772:bool)
                                n165 = Not(x=w776) -> (.not. x?=w777:bool)
                                n166 = Or(x=w772, y=w773) -> (x .or. y?=w771:bool)
                                n167 = case shown="True" w771 {
                                tunnel: w778 -> [_ w779]
                                frame False {
                                }
                                frame True {
                                n168 = VISA Write(VISA resource name=w779, write buffer="la off\r" ("format string")) -> ()  [unwired: 1 in, 3 out]
                                }
                                }
                                n169 = property on="odd/even indicator" class="Bool (strict)"("Value"=w777) -> ()  [unwired: 2 in, 2 out]
                                }
                                }
                              }
                            }
                            n170 = case shown="True" "acquire 561" {
                              tunnel: w469 -> [w617 w628]
                              tunnel: w468 -> [w618 w629]
                              tunnel: [w616 w626] -> w465
                              tunnel: [w618 w627] -> w464
                              tunnel: [w617 w625] -> w463
                              tunnel: w467 -> [w616 w624]
                              tunnel: w461 -> [_ _]
                              tunnel: w454 -> [_ w621]
                              tunnel: w458 -> [_ w620]
                              tunnel: w451 -> [_ w619]
                              frame False {
                              }
                              frame True {
                                n171 = property on="561 voltages" class="Arr (strict)"() -> ("Value"=w622:dbl[][])  [unwired: 2 in, 2 out]
                                n172 = stacked-sequence {
                                seq-local: [_ w639 _ _] -> [_ _ w661 _]
                                seq-local: [_ w638 _ _] -> [_ _ w660 _]
                                seq-local: [_ w637 _ _] -> [_ _ w656 _]
                                seq-local: [_ w636 _ _] -> [_ _ w654 _]
                                seq-local: [_ w635 _ _] -> [_ _ w653 _]
                                tunnel: w629 -> [_ w639 _ _]
                                tunnel: w628 -> [_ w638 _ _]
                                tunnel: w624 -> [_ w637 _ _]
                                tunnel: w622 -> [_ w636 _ _]
                                tunnel: "561 Exp" -> [_ w635 _ _]
                                tunnel: [_ _ w659 _] -> w627
                                tunnel: [_ _ w658 _] -> w626
                                tunnel: [_ _ w657 _] -> w625
                                tunnel: w622 -> [_ w633 _ _]
                                tunnel: w621 -> [_ w632 _ _]
                                tunnel: w620 -> [w631 _ _ w695]
                                tunnel: w619 -> [_ _ w652 _]
                                frame #0 {
                                n173 = call-poly <vilib>:"DAQmx Write.vi"("task/channels in"=w631, "data"=TRUE) -> ()  [unwired: 11 in, 3 out]
                                }
                                frame #1 {
                                n174 = flat-sequence {
                                tunnel: w633 -> [w643]
                                tunnel: [w642] -> w634
                                tunnel: w632 -> [w641]
                                tunnel: [w651] -> _
                                tunnel: w634 -> [w651]
                                frame #0 {
                                n175 = property on="odd/even indicator" class="Bool (strict)"() -> ("Value"=w640:bool)  [unwired: 2 in, 2 out]
                                n176 = case shown="True" w640 {
                                tunnel: [2 0] -> w646
                                tunnel: [2 0] -> w645
                                frame False {
                                }
                                frame True {
                                }
                                }
                                n177 = Index Array(array=w643, index (row)=w646, index (col)=w645) -> (element=w644:dbl)
                                n178 = call-poly <vilib>:"DAQmx Write.vi"("task/channels in"=w641, "data"=w644) -> ("task out"=w642:refnum<k21>)  [unwired: 11 in, 2 out]
                                }
                                frame #1 {
                                }
                                }
                                }
                                frame #2 {
                                n179 = for {
                                N: 9 -> [_]
                                tunnel: w654 -> [w673]
                                tunnel: w656 -> [w670]
                                tunnel: w661 -> [w671]
                                tunnel: w660 -> [w669]
                                tunnel: w653 -> [w672]
                                tunnel: [w671] -> w659
                                tunnel: [w670] -> w658
                                tunnel: [w669] -> w657
                                tunnel: w652 -> [w662]
                                i -> [w666]
                                n180 = property on="odd/even indicator" class="Bool (strict)"() -> ("Value"=w663:bool)  [unwired: 2 in, 2 out]
                                n181 = case shown="False" w663 {
                                tunnel: [i32[] [2, 2, 1, 1, 1, 0, 0, 0, 0, 2, 2, 2, 2, 2, 0] i32[] [0, 0, 1, 1, 1, 2, 2, 2, 2, 2, 2, 2, 2, 2, 0]] -> w668
                                tunnel: [i32[] [1, 0, 2, 1, 0, 2, 1, 0, 0, 0, 1, 2, 3, 4, 0] i32[] [1, 2, 0, 1, 2, 0, 1, 2, 2, 0, 1, 2, 3, 4, 0]] -> w667
                                frame False {
                                }
                                frame True {
                                }
                                }
                                n182 = flat-sequence {
                                tunnel: w673 -> [w682]
                                tunnel: w672 -> [w686]
                                tunnel: w671 -> [w685]
                                tunnel: w670 -> [w684]
                                tunnel: w669 -> [w683]
                                tunnel: w665 -> [w680]
                                tunnel: w664 -> [w679]
                                tunnel: w662 -> [w678]
                                frame #0 {
                                n183 = Index Array(array=w682, index (row)=w680, index (col)=w679) -> (element=w681:dbl)
                                n184 = call "take image.vi"("Voltage"=w681, "Exposure time"=w686, "expose any"=w678, "Busy out"=w683, "Exp In"=w684, "Galvo"=w685) -> ()  [unwired: 6 in]
                                }
                                frame #1 {
                                n185 = property on="Delay time" class="DigNum (strict)"() -> ("Value"=w687:u32)  [unwired: 2 in, 2 out]
                                n186 = Wait (ms)(milliseconds to wait=w687) -> ()  [unwired: 1 out]
                                }
                                }
                                n187 = Index Array(array=w667, index=w666) -> (element=w665:i32)
                                n188 = Index Array(array=w668, index=w666) -> (element=w664:i32)
                                }
                                }
                                frame #3 {
                                n189 = property on="acquire 488" class="Bool (strict)"() -> ("Value"=w691:bool)  [unwired: 2 in, 2 out]
                                n190 = property on="acquire 405" class="Bool (strict)"() -> ("Value"=w692:bool)  [unwired: 2 in, 2 out]
                                n191 = property on="acquire 640" class="Bool (strict)"() -> ("Value"=w690:bool)  [unwired: 2 in, 2 out]
                                n192 = Or(x=w691, y=w692) -> (x .or. y?=w689:bool)
                                n193 = Or(x=w689, y=w690) -> (x .or. y?=w688:bool)
                                n194 = case shown="False" w688 {
                                tunnel: w695 -> [_ w696]
                                frame False {
                                }
                                frame True {
                                n195 = call-poly <vilib>:"DAQmx Write.vi"("task/channels in"=w696, "data"=FALSE) -> ()  [unwired: 11 in, 3 out]
                                }
                                }
                                n196 = property on="odd/even indicator" class="Bool (strict)"() -> ("Value"=w694:bool)  [unwired: 2 in, 2 out]
                                n197 = Not(x=w694) -> (.not. x?=w693:bool)
                                n198 = property on="odd/even indicator" class="Bool (strict)"("Value"=w693) -> ()  [unwired: 2 in, 2 out]
                                }
                                }
                              }
                            }
                            n199 = case shown="True" "acquire 488" {
                              tunnel: w465 -> [w538 w544]
                              tunnel: w463 -> [w536 w548]
                              tunnel: w464 -> [w537 w549]
                              tunnel: [w538 w546] -> _
                              tunnel: [w537 w547] -> _
                              tunnel: [w536 w545] -> _
                              tunnel: w460 -> [_ _]
                              tunnel: w454 -> [_ w541]
                              tunnel: w457 -> [_ w540]
                              tunnel: w451 -> [_ w539]
                              frame False {
                              }
                              frame True {
                                n200 = property on="488 voltages" class="Arr (strict)"() -> ("Value"=w542:dbl[][])  [unwired: 2 in, 2 out]
                                n201 = stacked-sequence {
                                seq-local: [_ w558 _ _] -> [_ _ w579 _]
                                seq-local: [_ w557 _ _] -> [_ _ w578 _]
                                seq-local: [_ w556 _ _] -> [_ _ w574 _]
                                seq-local: [_ w555 _ _] -> [_ _ w572 _]
                                seq-local: [_ w554 _ _] -> [_ _ w571 _]
                                tunnel: w549 -> [_ w558 _ _]
                                tunnel: w548 -> [_ w557 _ _]
                                tunnel: w544 -> [_ w556 _ _]
                                tunnel: w542 -> [_ w555 _ _]
                                tunnel: "488 Exp" -> [_ w554 _ _]
                                tunnel: [_ _ w577 _] -> w547
                                tunnel: [_ _ w576 _] -> w546
                                tunnel: [_ _ w575 _] -> w545
                                tunnel: w542 -> [_ w553 _ _]
                                tunnel: w541 -> [_ w552 _ _]
                                tunnel: w540 -> [w550 _ _ w613]
                                tunnel: w539 -> [_ _ w570 _]
                                frame #0 {
                                n202 = call-poly <vilib>:"DAQmx Write.vi"("task/channels in"=w550, "data"=TRUE) -> ()  [unwired: 11 in, 3 out]
                                }
                                frame #1 {
                                n203 = flat-sequence {
                                tunnel: w553 -> [w565]
                                tunnel: w552 -> [w563]
                                tunnel: [w564] -> _
                                frame #0 {
                                n204 = property on="odd/even indicator" class="Bool (strict)"() -> ("Value"=w559:bool)  [unwired: 2 in, 2 out]
                                n205 = case shown="False" w559 {
                                tunnel: [2 0] -> w561
                                tunnel: [2 0] -> w560
                                frame False {
                                }
                                frame True {
                                }
                                }
                                n206 = Index Array(array=w565, index (row)=w561, index (col)=w560) -> (element=w562:dbl)
                                n207 = call-poly <vilib>:"DAQmx Write.vi"("task/channels in"=w563, "data"=w562) -> ("task out"=w564:refnum<k21>)  [unwired: 11 in, 2 out]
                                }
                                }
                                }
                                frame #2 {
                                n208 = for {
                                N: 9 -> [_]
                                tunnel: w572 -> [w591]
                                tunnel: w574 -> [w589]
                                tunnel: w579 -> [w590]
                                tunnel: w578 -> [w588]
                                tunnel: [w590] -> w577
                                tunnel: [w589] -> w576
                                tunnel: [w588] -> w575
                                tunnel: w571 -> [w587]
                                tunnel: w570 -> [w580]
                                i -> [w586]
                                n209 = property on="odd/even indicator" class="Bool (strict)"() -> ("Value"=w581:bool)  [unwired: 2 in, 2 out]
                                n210 = case shown="True" w581 {
                                tunnel: [i32[] [2, 2, 1, 1, 1, 0, 0, 0, 0, 2, 2, 2, 2, 2, 0] i32[] [0, 0, 1, 1, 1, 2, 2, 2, 2, 2, 2, 2, 2, 2, 0]] -> w582
                                tunnel: [i32[] [1, 0, 2, 1, 0, 2, 1, 0, 0, 0, 1, 2, 3, 4, 0] i32[] [1, 2, 0, 1, 2, 0, 1, 2, 2, 0, 1, 2, 3, 4, 0]] -> w583
                                frame False {
                                }
                                frame True {
                                }
                                }
                                n211 = Index Array(array=w583, index=w586) -> (element=w585:i32)
                                n212 = Index Array(array=w582, index=w586) -> (element=w584:i32)
                                n213 = flat-sequence {
                                tunnel: w591 -> [w600]
                                tunnel: w587 -> [w604]
                                tunnel: w590 -> [w603]
                                tunnel: w589 -> [w602]
                                tunnel: w588 -> [w601]
                                tunnel: w585 -> [w598]
                                tunnel: w584 -> [w597]
                                tunnel: w580 -> [w596]
                                frame #0 {
                                n214 = Index Array(array=w600, index (row)=w598, index (col)=w597) -> (element=w599:dbl)
                                n215 = call "take image.vi"("Voltage"=w599, "Exposure time"=w604, "expose any"=w596, "Busy out"=w601, "Exp In"=w602, "Galvo"=w603) -> ()  [unwired: 6 in]
                                }
                                frame #1 {
                                n216 = property on="Delay time" class="DigNum (strict)"() -> ("Value"=w605:u32)  [unwired: 2 in, 2 out]
                                n217 = Wait (ms)(milliseconds to wait=w605) -> ()  [unwired: 1 out]
                                }
                                }
                                }
                                }
                                frame #3 {
                                n218 = property on="acquire 561" class="Bool (strict)"() -> ("Value"=w609:bool)  [unwired: 2 in, 2 out]
                                n219 = property on="acquire 405" class="Bool (strict)"() -> ("Value"=w608:bool)  [unwired: 2 in, 2 out]
                                n220 = property on="acquire 640" class="Bool (strict)"() -> ("Value"=w610:bool)  [unwired: 2 in, 2 out]
                                n221 = property on="odd/even indicator" class="Bool (strict)"() -> ("Value"=w611:bool)  [unwired: 2 in, 2 out]
                                n222 = Not(x=w611) -> (.not. x?=w612:bool)
                                n223 = Or(x=w609, y=w608) -> (x .or. y?=w607:bool)
                                n224 = property on="odd/even indicator" class="Bool (strict)"("Value"=w612) -> ()  [unwired: 2 in, 2 out]
                                n225 = Or(x=w607, y=w610) -> (x .or. y?=w606:bool)
                                n226 = case shown="True" w606 {
                                tunnel: w613 -> [_ w614]
                                frame False {
                                }
                                frame True {
                                n227 = call-poly <vilib>:"DAQmx Write.vi"("task/channels in"=w614, "data"=FALSE) -> ()  [unwired: 11 in, 3 out]
                                }
                                }
                                }
                                }
                              }
                            }
                            n228 = case shown="True" "acquire 405" {
                              tunnel: w456 -> [_ w479]
                              tunnel: w454 -> [_ w477]
                              tunnel: w453 -> [_ w475]
                              tunnel: w452 -> [_ w474]
                              tunnel: w451 -> [_ w473]
                              frame False {
                              }
                              frame True {
                                n229 = property on="405 voltages" class="Arr (strict)"() -> ("Value"=w478:dbl[][])  [unwired: 2 in, 2 out]
                                n230 = stacked-sequence {
                                tunnel: w478 -> [_ w483 w498 _]
                                tunnel: w477 -> [_ w482 w497 _]
                                tunnel: [_ _ _ w533] -> _
                                tunnel: w479 -> [w480 _ _ w533]
                                tunnel: "405 Exp" -> [_ _ w496 _]
                                tunnel: w475 -> [_ _ w495 _]
                                tunnel: w474 -> [_ _ w494 _]
                                tunnel: w473 -> [_ _ w493 _]
                                frame #0 {
                                n231 = call-poly <vilib>:"DAQmx Write.vi"("task/channels in"=w480, "data"=TRUE) -> ()  [unwired: 11 in, 3 out]
                                }
                                frame #1 {
                                n232 = flat-sequence {
                                tunnel: w483 -> [w487]
                                tunnel: [w486] -> w484
                                tunnel: w482 -> [w485]
                                tunnel: [w492] -> _
                                tunnel: w484 -> [w492]
                                frame #0 {
                                n233 = Index Array(array=w487, index (row)=0, index (col)=0) -> (element=w488:dbl)
                                n234 = call-poly <vilib>:"DAQmx Write.vi"("task/channels in"=w485, "data"=w488) -> ("task out"=w486:refnum<k21>)  [unwired: 11 in, 2 out]
                                }
                                frame #1 {
                                n235 = Wait (ms)(milliseconds to wait=50) -> ()  [unwired: 1 out]
                                }
                                }
                                }
                                frame #2 {
                                n236 = for {
                                N: 9 -> [_]
                                tunnel: w498 -> [w509]
                                tunnel: w497 -> [w508]
                                tunnel: w496 -> [w507]
                                tunnel: w495 -> [w506]
                                tunnel: w494 -> [w505]
                                tunnel: w493 -> [w500]
                                i -> [w504]
                                n237 = property on="odd/even indicator" class="Bool (strict)"() -> ("Value"=w501:bool)  [unwired: 2 in, 2 out]
                                n238 = case shown="True" w501 {
                                tunnel: [i32[] [2, 2, 1, 1, 1, 0, 0, 0, 0, 2, 2, 2, 2, 2, 0] i32[] [0, 0, 1, 1, 1, 2, 2, 2, 2, 2, 2, 2, 2, 2, 0]] -> w503
                                tunnel: [i32[] [1, 0, 2, 1, 0, 2, 1, 0, 0, 0, 1, 2, 3, 4, 0] i32[] [1, 2, 0, 1, 2, 0, 1, 2, 2, 0, 1, 2, 3, 4, 0]] -> w502
                                frame False {
                                }
                                frame True {
                                }
                                }
                                n239 = flat-sequence {
                                tunnel: w511 -> [w523]
                                tunnel: w510 -> [w522]
                                tunnel: w509 -> [w521]
                                tunnel: w508 -> [w520]
                                tunnel: w507 -> [w519]
                                tunnel: w506 -> [w518]
                                tunnel: w505 -> [w517]
                                tunnel: w500 -> [w516]
                                frame #0 {
                                n240 = Index Array(array=w521, index (row)=w523, index (col)=w522) -> (element=w524:dbl)
                                n241 = call "take image.vi"("Voltage"=w524, "Exposure time"=w519, "expose any"=w516, "Busy out"=w517, "Exp In"=w518, "Galvo"=w520) -> ()  [unwired: 6 in]
                                }
                                frame #1 {
                                n242 = property on="Delay time" class="DigNum (strict)"() -> ("Value"=w525:u32)  [unwired: 2 in, 2 out]
                                n243 = Wait (ms)(milliseconds to wait=w525) -> ()  [unwired: 1 out]
                                }
                                }
                                n244 = Index Array(array=w502, index=w504) -> (element=w511:i32)
                                n245 = Index Array(array=w503, index=w504) -> (element=w510:i32)
                                }
                                }
                                frame #3 {
                                n246 = property on="acquire 561" class="Bool (strict)"() -> ("Value"=w528:bool)  [unwired: 2 in, 2 out]
                                n247 = property on="acquire 488" class="Bool (strict)"() -> ("Value"=w529:bool)  [unwired: 2 in, 2 out]
                                n248 = property on="acquire 640" class="Bool (strict)"() -> ("Value"=w527:bool)  [unwired: 2 in, 2 out]
                                n249 = Or(x=w528, y=w529) -> (x .or. y?=w530:bool)
                                n250 = property on="odd/even indicator" class="Bool (strict)"() -> ("Value"=w532:bool)  [unwired: 2 in, 2 out]
                                n251 = Or(x=w530, y=w527) -> (x .or. y?=w526:bool)
                                n252 = Not(x=w532) -> (.not. x?=w531:bool)
                                n253 = property on="odd/even indicator" class="Bool (strict)"("Value"=w531) -> ()  [unwired: 2 in, 2 out]
                                n254 = case shown="True" w526 {
                                tunnel: w533 -> [_ w534]
                                frame False {
                                }
                                frame True {
                                n255 = call-poly <vilib>:"DAQmx Write.vi"("task/channels in"=w534, "data"=FALSE) -> ()  [unwired: 11 in, 3 out]
                                }
                                }
                                }
                                }
                              }
                            }
                          }
                          frame "fast sequence" {
                            # "561"
                            # "488"
                            # "fast sequence"
                            n256 = property on="647 Exp" class="DigNum (strict)"() -> ("Value"=w784:dbl)  [unwired: 2 in, 2 out]
                            n257 = property on="647 voltages" class="Arr (strict)"() -> ("Value"=w787:dbl[][])  [unwired: 2 in, 2 out]
                            n258 = stacked-sequence {
                              seq-local: [_ w869 _ _] -> [_ _ w887 _]
                              seq-local: [_ w868 _ _] -> [_ _ w886 _]
                              seq-local: [_ w867 _ _] -> [_ _ w885 _]
                              seq-local: [_ w866 _ _] -> [_ _ w881 _]
                              seq-local: [_ w865 _ _] -> [_ _ w880 _]
                              tunnel: w795 -> [_ w869 _ _]
                              tunnel: w790 -> [_ w868 _ _]
                              tunnel: w794 -> [_ w867 _ _]
                              tunnel: w787 -> [_ w866 _ _]
                              tunnel: w784 -> [_ w865 _ _]
                              tunnel: [_ _ w884 _] -> w792
                              tunnel: [_ _ w883 _] -> w791
                              tunnel: [_ _ w882 _] -> w793
                              tunnel: w787 -> [_ w863 _ _]
                              tunnel: w790 -> [_ w862 _ _]
                              tunnel: w789 -> [w860 _ _ w918]
                              tunnel: w783 -> [w858 _ _ w916]
                              tunnel: w781 -> [_ _ w878 _]
                              frame #0 {
                                n259 = VISA Write(VISA resource name=w860, write buffer="la on\r" ("format string")) -> ()  [unwired: 1 in, 3 out]
                                n260 = call-poly <vilib>:"DAQmx Write.vi"("task/channels in"=w858, "data"=TRUE) -> ()  [unwired: 11 in, 3 out]
                              }
                              frame #1 {
                                n261 = flat-sequence {
                                tunnel: [w870] -> _
                                tunnel: w863 -> [w872]
                                tunnel: [w871] -> w864
                                tunnel: w862 -> [w870]
                                tunnel: [w877] -> _
                                tunnel: w864 -> [w877]
                                frame #0 {
                                n262 = Index Array(array=w872, index (row)=0, index (col)=0) -> (element=w873:dbl)
                                n263 = call-poly <vilib>:"DAQmx Write.vi"("task/channels in"=w870, "data"=w873) -> ("task out"=w871:refnum<k21>)  [unwired: 11 in, 2 out]
                                }
                                frame #1 {
                                n264 = Wait (ms)(milliseconds to wait=50) -> ()  [unwired: 1 out]
                                }
                                }
                              }
                              frame #2 {
                                n265 = for {
                                N: 9 -> [_]
                                tunnel: w881 -> [w899]
                                tunnel: w887 -> [w896]
                                tunnel: w886 -> [w897]
                                tunnel: w885 -> [w895]
                                tunnel: w880 -> [w898]
                                tunnel: [w897] -> w884
                                tunnel: [w896] -> w883
                                tunnel: [w895] -> w882
                                tunnel: w878 -> [w888]
                                i -> [w893]
                                n266 = property on="odd/even indicator" class="Bool (strict)"() -> ("Value"=w891:bool)  [unwired: 2 in, 2 out]
                                n267 = case shown="False" w891 {
                                tunnel: [i32[] [2, 2, 1, 1, 1, 0, 0, 0, 0, 2, 2, 2, 2, 2, 0] i32[] [0, 0, 1, 1, 1, 2, 2, 2, 2, 2, 2, 2, 2, 2, 0]] -> w889
                                tunnel: [i32[] [1, 0, 2, 1, 0, 2, 1, 0, 0, 0, 1, 2, 3, 4, 0] i32[] [1, 2, 0, 1, 2, 0, 1, 2, 2, 0, 1, 2, 3, 4, 0]] -> w890
                                frame False {
                                }
                                frame True {
                                }
                                }
                                n268 = Index Array(array=w890, index=w893) -> (element=w894:i32)
                                n269 = flat-sequence {
                                tunnel: w899 -> [w908]
                                tunnel: w898 -> [w912]
                                tunnel: w897 -> [w911]
                                tunnel: w896 -> [w910]
                                tunnel: w895 -> [w909]
                                tunnel: w892 -> [w906]
                                tunnel: w894 -> [w905]
                                tunnel: w888 -> [w904]
                                frame #0 {
                                n270 = Index Array(array=w908, index (row)=w905, index (col)=w906) -> (element=w907:dbl)
                                n271 = call "take image.vi"("Voltage"=w907, "Exposure time"=w912, "expose any"=w904, "Busy out"=w909, "Exp In"=w910, "Galvo"=w911) -> ()  [unwired: 6 in]
                                }
                                frame #1 {
                                n272 = property on="Delay time" class="DigNum (strict)"() -> ("Value"=w913:u32)  [unwired: 2 in, 2 out]
                                n273 = Wait (ms)(milliseconds to wait=w913) -> ()  [unwired: 1 out]
                                }
                                }
                                n274 = Index Array(array=w889, index=w893) -> (element=w892:i32)
                                }
                              }
                              frame #3 {
                                n275 = property on="odd/even indicator" class="Bool (strict)"() -> ("Value"=w914:bool)  [unwired: 2 in, 2 out]
                                n276 = Not(x=w914) -> (.not. x?=w915:bool)
                                n277 = property on="odd/even indicator" class="Bool (strict)"("Value"=w915) -> ()  [unwired: 2 in, 2 out]
                                n278 = VISA Write(VISA resource name=w918, write buffer="la off\r" ("format string")) -> ()  [unwired: 1 in, 3 out]
                                n279 = call-poly <vilib>:"DAQmx Write.vi"("task/channels in"=w916, "data"=FALSE) -> ()  [unwired: 11 in, 3 out]
                              }
                            }
                            n280 = property on="561 voltages" class="Arr (strict)"() -> ("Value"=w786:dbl[][])  [unwired: 2 in, 2 out]
                            n281 = property on="561 Exp" class="DigNum (strict)"() -> ("Value"=w785:dbl)  [unwired: 2 in, 2 out]
                            n282 = stacked-sequence {
                              seq-local: [_ w807 _ _] -> [_ _ w825 _]
                              seq-local: [_ w806 _ _] -> [_ _ w824 _]
                              seq-local: [_ w805 _ _] -> [_ _ w820 _]
                              seq-local: [_ w804 _ _] -> [_ _ w818 _]
                              seq-local: [_ w803 _ _] -> [_ _ w817 _]
                              tunnel: w792 -> [_ w807 _ _]
                              tunnel: w793 -> [_ w806 _ _]
                              tunnel: w791 -> [_ w805 _ _]
                              tunnel: w786 -> [_ w804 _ _]
                              tunnel: w785 -> [_ w803 _ _]
                              tunnel: [_ _ w823 _] -> _
                              tunnel: [_ _ w822 _] -> _
                              tunnel: [_ _ w821 _] -> _
                              tunnel: w786 -> [_ w801 _ _]
                              tunnel: w790 -> [_ w800 _ _]
                              tunnel: w788 -> [w799 _ _ w856]
                              tunnel: w782 -> [w796 _ _ w854]
                              tunnel: w781 -> [_ _ w816 _]
                              frame #0 {
                                n283 = call-poly <vilib>:"DAQmx Write.vi"("task/channels in"=w799, "data"=TRUE) -> ()  [unwired: 11 in, 3 out]
                                n284 = call-poly <vilib>:"DAQmx Write.vi"("task/channels in"=w796, "data"=TRUE) -> ()  [unwired: 11 in, 3 out]
                              }
                              frame #1 {
                                n285 = flat-sequence {
                                tunnel: w801 -> [w810]
                                tunnel: [w809] -> w802
                                tunnel: w800 -> [w808]
                                tunnel: [w815] -> _
                                tunnel: w802 -> [w815]
                                frame #0 {
                                n286 = Index Array(array=w810, index (row)=0, index (col)=0) -> (element=w811:dbl)
                                n287 = call-poly <vilib>:"DAQmx Write.vi"("task/channels in"=w808, "data"=w811) -> ("task out"=w809:refnum<k21>)  [unwired: 11 in, 2 out]
                                }
                                frame #1 {
                                n288 = Wait (ms)(milliseconds to wait=50) -> ()  [unwired: 1 out]
                                }
                                }
                              }
                              frame #2 {
                                n289 = for {
                                N: 9 -> [_]
                                tunnel: w818 -> [w837]
                                tunnel: w820 -> [w834]
                                tunnel: w825 -> [w835]
                                tunnel: w824 -> [w833]
                                tunnel: w817 -> [w836]
                                tunnel: [w835] -> w823
                                tunnel: [w834] -> w822
                                tunnel: [w833] -> w821
                                tunnel: w816 -> [w826]
                                i -> [w832]
                                n290 = property on="odd/even indicator" class="Bool (strict)"() -> ("Value"=w827:bool)  [unwired: 2 in, 2 out]
                                n291 = case shown="True" w827 {
                                tunnel: [i32[] [2, 2, 1, 1, 1, 0, 0, 0, 0, 2, 2, 2, 2, 2, 0] i32[] [0, 0, 1, 1, 1, 2, 2, 2, 2, 2, 2, 2, 2, 2, 0]] -> w828
                                tunnel: [i32[] [1, 0, 2, 1, 0, 2, 1, 0, 0, 0, 1, 2, 3, 4, 0] i32[] [1, 2, 0, 1, 2, 0, 1, 2, 2, 0, 1, 2, 3, 4, 0]] -> w829
                                frame False {
                                }
                                frame True {
                                }
                                }
                                n292 = Index Array(array=w829, index=w832) -> (element=w831:i32)
                                n293 = Index Array(array=w828, index=w832) -> (element=w830:i32)
                                n294 = flat-sequence {
                                tunnel: w837 -> [w846]
                                tunnel: w836 -> [w850]
                                tunnel: w835 -> [w849]
                                tunnel: w834 -> [w848]
                                tunnel: w833 -> [w847]
                                tunnel: w831 -> [w844]
                                tunnel: w830 -> [w843]
                                tunnel: w826 -> [w842]
                                frame #0 {
                                n295 = Index Array(array=w846, index (row)=w844, index (col)=w843) -> (element=w845:dbl)
                                n296 = call "take image.vi"("Voltage"=w845, "Exposure time"=w850, "expose any"=w842, "Busy out"=w847, "Exp In"=w848, "Galvo"=w849) -> ()  [unwired: 6 in]
                                }
                                frame #1 {
                                n297 = property on="Delay time" class="DigNum (strict)"() -> ("Value"=w851:u32)  [unwired: 2 in, 2 out]
                                n298 = Wait (ms)(milliseconds to wait=w851) -> ()  [unwired: 1 out]
                                }
                                }
                                }
                              }
                              frame #3 {
                                n299 = call-poly <vilib>:"DAQmx Write.vi"("task/channels in"=w856, "data"=FALSE) -> ()  [unwired: 11 in, 3 out]
                                n300 = property on="odd/even indicator" class="Bool (strict)"() -> ("Value"=w853:bool)  [unwired: 2 in, 2 out]
                                n301 = call-poly <vilib>:"DAQmx Write.vi"("task/channels in"=w854, "data"=FALSE) -> ()  [unwired: 11 in, 3 out]
                                n302 = Not(x=w853) -> (.not. x?=w852:bool)
                                n303 = property on="odd/even indicator" class="Bool (strict)"("Value"=w852) -> ()  [unwired: 2 in, 2 out]
                              }
                            }
                          }
                          frame "optosplit" {
                            n304 = case shown="False" w921 {
                              tunnel: w924 -> [w930 w967]
                              tunnel: w923 -> [w929 w966]
                              tunnel: w922 -> [w928 w965]
                              tunnel: w920 -> [_ w959]
                              frame True {
                                w925 = 15
                                # "With optosplit"
                                n305 = flat-sequence {
                                tunnel: w928 -> [w934]
                                tunnel: w927 -> [w933]
                                tunnel: [w932] -> w931
                                tunnel: [w941] -> w926
                                tunnel: w931 -> [w941]
                                frame #0 {
                                n306 = Index Array(array=w933, index (row)=0, index (col)=0) -> (element=w935:dbl)
                                n307 = call-poly <vilib>:"DAQmx Write.vi"("task/channels in"=w934, "data"=w935) -> ("task out"=w932:refnum<k21>)  [unwired: 11 in, 2 out]
                                }
                                frame #1 {
                                n308 = property on="Delay time" class="DigNum (strict)"() -> ("Value"=w940:u32)  [unwired: 2 in, 2 out]
                                n309 = Add(x=w940, y=20) -> (x+y=w939:u32)
                                n310 = Wait (ms)(milliseconds to wait=w939) -> ()  [unwired: 1 out]
                                }
                                }
                                n311 = property on="561 voltages" class="Arr (strict)"() -> ("Value"=w927:dbl[][])  [unwired: 2 in, 2 out]
                                n312 = for {
                                N: w925 -> [_]
                                tunnel: w927 -> [w949]
                                tunnel: w930 -> [w952]
                                tunnel: w929 -> [w951]
                                tunnel: w926 -> [w950]
                                tunnel: w925 -> [_]
                                i -> [w945]
                                n313 = property on="Exposure \n(ms)" class="DigNum (strict)"() -> ("Value"=w948:dbl)  [unwired: 2 in, 2 out]
                                n314 = Index Array(array=i32[] [1, 2, 3, 4, 0, 1, 2, 3, 4, 0, 1, 2, 3, 4, 0], index=w945) -> (element=w943:i32)
                                n315 = Index Array(array=i32[] [0, 0, 0, 0, 1, 1, 1, 1, 1, 2, 2, 2, 2, 2, 0], index=w945) -> (element=w944:i32)
                                n316 = Index Array(array=w949, index (row)=w943, index (col)=w944) -> (element=w942:dbl)
                                n317 = property on="Current voltage" class="DigNum (strict)"("Value"=w942) -> ()  [unwired: 2 in, 2 out]
                                n318 = flat-sequence {
                                tunnel: w952 -> [w957]
                                tunnel: w951 -> [w956]
                                tunnel: w942 -> [w955]
                                tunnel: w950 -> [w954]
                                tunnel: w948 -> [w953]
                                frame #0 {
                                n319 = call "take image.vi"("Voltage"=w955, "Exposure time"=w953, "Busy out"=w956, "Exp In"=w957, "Galvo"=w954) -> ()  [unwired: 7 in]
                                }
                                frame #1 {
                                n320 = property on="Delay time" class="DigNum (strict)"() -> ("Value"=w958:u32)  [unwired: 2 in, 2 out]
                                n321 = Wait (ms)(milliseconds to wait=w958) -> ()  [unwired: 1 out]
                                }
                                }
                                }
                              }
                              frame False {
                                w962 = 9
                                # "With optosplit"
                                n322 = flat-sequence {
                                tunnel: w965 -> [w974]
                                tunnel: w964 -> [w973]
                                tunnel: [w972] -> w968
                                tunnel: [w983] -> w963
                                tunnel: w968 -> [w983]
                                frame #0 {
                                n323 = property on="odd/even indicator" class="Bool (strict)"() -> ("Value"=w971:bool)  [unwired: 2 in, 2 out]
                                n324 = case shown="False" w971 {
                                tunnel: [2 0] -> w970
                                tunnel: [2 0] -> w969
                                frame False {
                                }
                                frame True {
                                }
                                }
                                n325 = Index Array(array=w973, index (row)=w970, index (col)=w969) -> (element=w975:dbl)
                                n326 = call-poly <vilib>:"DAQmx Write.vi"("task/channels in"=w974, "data"=w975) -> ("task out"=w972:refnum<k21>)  [unwired: 11 in, 2 out]
                                }
                                frame #1 {
                                n327 = property on="Delay time" class="DigNum (strict)"() -> ("Value"=w982:u32)  [unwired: 2 in, 2 out]
                                n328 = Add(x=w982, y=20) -> (x+y=w981:u32)
                                n329 = Wait (ms)(milliseconds to wait=w981) -> ()  [unwired: 1 out]
                                }
                                }
                                n330 = property on="561 voltages" class="Arr (strict)"() -> ("Value"=w964:dbl[][])  [unwired: 2 in, 2 out]
                                n331 = for {
                                N: w962 -> [_]
                                tunnel: w964 -> [w993]
                                tunnel: w967 -> [w996]
                                tunnel: w966 -> [w995]
                                tunnel: w963 -> [w994]
                                tunnel: w962 -> [_]
                                tunnel: [w985] -> w960
                                tunnel: w959 -> [w984]
                                i -> [w991]
                                n332 = property on="odd/even indicator" class="Bool (strict)"() -> ("Value"=w985:bool)  [unwired: 2 in, 2 out]
                                n333 = property on="Exposure \n(ms)" class="DigNum (strict)"() -> ("Value"=w992:dbl)  [unwired: 2 in, 2 out]
                                n334 = case shown="False" w985 {
                                tunnel: [i32[] [2, 2, 1, 1, 1, 0, 0, 0, 0, 2, 2, 2, 2, 2, 0] i32[] [0, 0, 1, 1, 1, 2, 2, 2, 2, 2, 2, 2, 2, 2, 0]] -> w986
                                tunnel: [i32[] [1, 0, 2, 1, 0, 2, 1, 0, 0, 0, 1, 2, 3, 4, 0] i32[] [1, 2, 0, 1, 2, 0, 1, 2, 2, 0, 1, 2, 3, 4, 0]] -> w987
                                frame False {
                                }
                                frame True {
                                }
                                }
                                n335 = Index Array(array=w987, index=w991) -> (element=w989:i32)
                                n336 = Index Array(array=w986, index=w991) -> (element=w990:i32)
                                n337 = Index Array(array=w993, index (row)=w989, index (col)=w990) -> (element=w988:dbl)
                                n338 = property on="Current voltage" class="DigNum (strict)"("Value"=w988) -> ()  [unwired: 2 in, 2 out]
                                n339 = flat-sequence {
                                tunnel: w996 -> [w1006]
                                tunnel: w995 -> [w1005]
                                tunnel: w988 -> [w1004]
                                tunnel: w994 -> [w1003]
                                tunnel: w992 -> [w1002]
                                tunnel: w984 -> [w1001]
                                frame #0 {
                                n340 = call "take image.vi"("Voltage"=w1004, "Exposure time"=w1002, "expose any"=w1001, "Busy out"=w1005, "Exp In"=w1006, "Galvo"=w1003) -> ()  [unwired: 6 in]
                                }
                                frame #1 {
                                n341 = property on="Delay time" class="DigNum (strict)"() -> ("Value"=w1007:u32)  [unwired: 2 in, 2 out]
                                n342 = Wait (ms)(milliseconds to wait=w1007) -> ()  [unwired: 1 out]
                                }
                                }
                                }
                                n343 = Not(x=w960) -> (.not. x?=w961:bool)
                                n344 = property on="odd/even indicator" class="Bool (strict)"("Value"=w961) -> ()  [unwired: 2 in, 2 out]
                              }
                            }
                          }
                          frame "rolling SIM" {
                            w1011 = 0 ("index")
                            # "Rolling SIM"
                            n345 = Build Array("short delay", "short delay", "long delay") -> (w1012:dbl[])
                            n346 = Insert Into Array(array=w1012, index=w1011, new element=w1012) -> (w1013:dbl[])
                            n347 = Insert Into Array(array=w1013, index=w1011, new element=w1013) -> (w1008:dbl[])
                            n348 = property on="561 voltages" class="Arr (strict)"() -> ("Value"=w1019:dbl[][])  [unwired: 2 in, 2 out]
                            n349 = for {
                              N: 12 -> [_]
                              tunnel: w1019 -> [w1024]
                              tunnel: w1021 -> [w1035]
                              tunnel: w1020 -> [w1034]
                              tunnel: [w1027] -> w1016
                              tunnel: w1015 -> [w1026]
                              tunnel: w1014 -> [w1025]
                              tunnel: w1008 -> [w1022] mode=indexing
                              i -> [w1023]
                              n350 = property on="Exposure \n(ms)" class="DigNum (strict)"() -> ("Value"=w1033:dbl)  [unwired: 2 in, 2 out]
                              n351 = Index Array(array=i32[] [1, 2, 0, 1, 2, 0, 1, 2, 2, 1, 0, 0, 3, 4, 0], index=w1023) -> (element=w1031:i32)
                              n352 = Index Array(array=i32[] [0, 0, 1, 1, 1, 2, 2, 2, 1, 1, 1, 0, 2, 2, 0], index=w1023) -> (element=w1032:i32)
                              n353 = Index Array(array=w1024, index (row)=w1031, index (col)=w1032) -> (element=w1030:dbl)
                              n354 = property on="Current voltage" class="DigNum (strict)"("Value"=w1030) -> ()  [unwired: 2 in, 2 out]
                              n355 = flat-sequence {
                                tunnel: w1035 -> [w1041]
                                tunnel: w1034 -> [w1037]
                                tunnel: w1030 -> [w1040]
                                tunnel: w1033 -> [w1039]
                                tunnel: w1026 -> [w1038]
                                tunnel: w1025 -> [w1036]
                                tunnel: w1022 -> [w1042]
                                frame #0 {
                                n356 = call "take image.vi"("Voltage"=w1040, "Exposure time"=w1039, "expose any"=w1038, "Busy out"=w1037, "Exp In"=w1041, "Galvo"=w1036) -> ()  [unwired: 6 in]
                                }
                                frame #1 {
                                n357 = Wait (ms)(milliseconds to wait=w1042) -> ()  [unwired: 1 out]
                                }
                              }
                              n358 = property on="odd/even indicator" class="Bool (strict)"() -> ("Value"=w1027:bool)  [unwired: 2 in, 2 out]
                            }
                            n359 = Not(x=w1016) -> (.not. x?=w1017:bool)
                            n360 = property on="odd/even indicator" class="Bool (strict)"("Value"=w1017) -> ()  [unwired: 2 in, 2 out]
                          }
                        }
                      }
                      frame #1 {
                        n361 = Greater?(x=w1046, y=1) -> (0:w1045:bool)
                        n362 = Greater?(x="Steps /um", y=0) -> (0:w1044:bool)
                        n363 = And(x=w1045, y=w1044) -> (x .and. y?=w1043:bool)
                        n364 = case shown="True" w1043 {
                          tunnel: w1051 -> [w1052 w1055]
                          tunnel: [w1052 w1054] -> w1050
                          tunnel: "Steps /um" -> [_ w1053]
                          frame False {
                          }
                          frame True {
                            n365 = flat-sequence {
                              tunnel: w1055 -> [w1063]
                              tunnel: [w1062] -> w1056
                              tunnel: w1053 -> [w1059]
                              tunnel: [w1066] -> w1054
                              tunnel: w1056 -> [w1066]
                              frame #0 {
                                n366 = Multiply(x=w1059, y=10.0) -> (x*y=w1057:dbl)
                                n367 = Format Into String "Format Into String"(format string="movrel\\sz=%f\\s\\r\\n", w1057) -> (resulting string=w1060:string)  [unwired: 2 in, 1 out]
                                "resulting string" <- w1060
                                n368 = VISA Write(VISA resource name=w1063, write buffer=w1060) -> (VISA resource name out=w1062:refnum<visa-resource-name>, error out=→"optosplit stage error":errorcluster)  [unwired: 1 in, 1 out]
                              }
                              frame #1 {
                                n369 = Wait (ms)(milliseconds to wait=20) -> ()  [unwired: 1 out]
                              }
                            }
                          }
                        }
                      }
                    }
                  }
                }
                frame #1 {
                  n370 = flat-sequence {
                    tunnel: w1082 -> [w1092]
                    tunnel: w1081 -> [w1091]
                    tunnel: w1080 -> [w1090]
                    tunnel: w1079 -> [w1089]
                    tunnel: [w1088] -> w1076
                    tunnel: [w1087] -> w1073
                    tunnel: [w1086] -> w1070
                    tunnel: [w1085] -> w1069
                    tunnel: w1083 -> [w1116]
                    tunnel: [w1115] -> w1077
                    tunnel: w1076 -> [w1115]
                    tunnel: [w1114] -> w1074
                    tunnel: w1073 -> [w1114]
                    tunnel: [w1113] -> w1071
                    tunnel: w1070 -> [w1113]
                    tunnel: w1069 -> [w1112]
                    tunnel: [w1112] -> w1067
                    tunnel: [w1130] -> w1078
                    tunnel: w1077 -> [w1130]
                    tunnel: [w1129] -> w1075
                    tunnel: w1074 -> [w1129]
                    tunnel: [w1128] -> w1072
                    tunnel: w1071 -> [w1128]
                    tunnel: [w1127] -> w1068
                    tunnel: w1067 -> [w1127]
                    tunnel: w1078 -> [w1137]
                    tunnel: w1075 -> [w1136]
                    tunnel: w1072 -> [w1135]
                    tunnel: w1068 -> [w1134]
                    frame #0 {
                      n371 = case shown="False" FALSE {
                        tunnel: w1092 -> [w1096 w1104]
                        tunnel: w1091 -> [w1095 w1103]
                        tunnel: w1090 -> [w1094 w1102]
                        tunnel: w1089 -> [w1093 w1101]
                        tunnel: [w1093 w1100] -> w1088
                        tunnel: [w1094 w1099] -> w1087
                        tunnel: [w1095 w1098] -> w1086
                        tunnel: [w1096 w1097] -> w1085
                        frame False {
                        }
                        frame True {
                          n372 = call-poly <vilib>:"DAQmx Write.vi"("task/channels in"=w1103, "data"=FALSE) -> ("task out"=w1098:refnum<k21>)  [unwired: 11 in, 2 out]
                          n373 = call-poly <vilib>:"DAQmx Write.vi"("task/channels in"=w1104, "data"=FALSE) -> ("task out"=w1097:refnum<k21>)  [unwired: 11 in, 2 out]
                          n374 = call-poly <vilib>:"DAQmx Write.vi"("task/channels in"=w1102, "data"=FALSE) -> ("task out"=w1099:refnum<k21>)  [unwired: 11 in, 2 out]
                          n375 = VISA Write(VISA resource name=w1101, write buffer="la off\r" ("format string")) -> (VISA resource name out=w1100:refnum<visa-resource-name>)  [unwired: 1 in, 2 out]
                        }
                      }
                    }
                    frame #1 {
                      n376 = property on="z-slices" class="DigNum (strict)"() -> ("Value"=w1110:dbl)  [unwired: 2 in, 2 out]
                      n377 = property on="Optosplit" class="RadioBtnsControl (strict)" props=["Value"]() -> ()  [unwired: 2 in, 3 out]
                      n378 = Greater?(x=w1110, y=1) -> (0:w1109:bool)
                      n379 = case shown="False" w1109 {
                        tunnel: w1116 -> [_ w1123]
                        frame False {
                        }
                        frame True {
                          n380 = property on="z-slices" class="DigNum (strict)"() -> ("Value"=w1121:dbl)  [unwired: 2 in, 2 out]
                          n381 = property on="Steps /um" class="DigNum (strict)"() -> ("Value"=w1122:dbl)  [unwired: 2 in, 2 out]
                          n382 = Negate(x=w1122) -> (-x=w1120:dbl)
                          n383 = Multiply(x=w1120, y=w1121) -> (x*y=w1119:dbl)
                          n384 = Multiply(x=w1119, y=10.0) -> (x*y=w1117:dbl)
                          n385 = Format Into String "Format Into String"(format string="movrel\\sz=%f\\s\\r\\n", w1117) -> (resulting string=w1125:string)  [unwired: 2 in, 1 out]
                          "resulting string 2" <- w1125
                          n386 = VISA Write(VISA resource name=w1123, write buffer=w1125) -> (error out=→"stage error":errorcluster)  [unwired: 1 in, 2 out]
                        }
                      }
                    }
                    frame #2 {
                      n387 = Multiply(x="interval /s", y=1000.0) -> (x*y=w1133:dbl)
                      n388 = Wait (ms)(milliseconds to wait=w1133) -> ()  [unwired: 1 out]
                    }
                    frame #3 {
                      n389 = property on="Optosplit" class="RadioBtnsControl (strict)"() -> ("Value"=w1138:T2)  [unwired: 2 in, 2 out]
                      n390 = disable-structure shown="Disabled" {
                        disable-tunnel: w1138 -> [w1143 _]
                        disable-tunnel: w1137 -> [w1142 _]
                        disable-tunnel: w1136 -> [w1141 _]
                        disable-tunnel: w1135 -> [w1140 _]
                        disable-tunnel: w1134 -> [w1139 _]
                        frame Disabled {
                          n391 = case shown="\"rolling SIM\"" w1143 {
                            tunnel: w1142 -> [_ w1147 w1155 w1163]
                            tunnel: w1141 -> [_ w1146 w1154 w1162]
                            tunnel: w1140 -> [_ w1145 w1153 w1161]
                            tunnel: w1139 -> [_ w1144 w1152 w1160]
                            frame "sequential", Default {
                            }
                            frame "optosplit" {
                              n392 = call-poly <vilib>:"DAQmx Write.vi"("task/channels in"=w1145, "data"=TRUE) -> ()  [unwired: 11 in, 3 out]
                              n393 = call-poly <vilib>:"DAQmx Write.vi"("task/channels in"=w1144, "data"=TRUE) -> ()  [unwired: 11 in, 3 out]
                              n394 = call-poly <vilib>:"DAQmx Write.vi"("task/channels in"=w1146, "data"=TRUE) -> ()  [unwired: 11 in, 3 out]
                              n395 = VISA Write(VISA resource name=w1147, write buffer="la on\r" ("format string")) -> ()  [unwired: 1 in, 3 out]
                            }
                            frame "rolling SIM" {
                              n396 = call-poly <vilib>:"DAQmx Write.vi"("task/channels in"=w1153, "data"=TRUE) -> ()  [unwired: 11 in, 3 out]
                              n397 = call-poly <vilib>:"DAQmx Write.vi"("task/channels in"=w1152, "data"=TRUE) -> ()  [unwired: 11 in, 3 out]
                              n398 = call-poly <vilib>:"DAQmx Write.vi"("task/channels in"=w1154, "data"=TRUE) -> ()  [unwired: 11 in, 3 out]
                              n399 = VISA Write(VISA resource name=w1155, write buffer="la on\r" ("format string")) -> ()  [unwired: 1 in, 3 out]
                            }
                            frame "fast sequence" {
                              n400 = call-poly <vilib>:"DAQmx Write.vi"("task/channels in"=w1161, "data"=TRUE) -> ()  [unwired: 11 in, 3 out]
                              n401 = call-poly <vilib>:"DAQmx Write.vi"("task/channels in"=w1160, "data"=TRUE) -> ()  [unwired: 11 in, 3 out]
                              n402 = call-poly <vilib>:"DAQmx Write.vi"("task/channels in"=w1162, "data"=TRUE) -> ()  [unwired: 11 in, 3 out]
                              n403 = VISA Write(VISA resource name=w1163, write buffer="la on\r" ("format string")) -> ()  [unwired: 1 in, 3 out]
                            }
                          }
                        }
                        frame Enabled {
                        }
                      }
                    }
                  }
                }
              }
              n404 = property on="Go SIM" class="Bool (strict)"() -> ("Value"=w383:bool)  [unwired: 2 in, 2 out]
              n405 = Not(x=w383) -> (.not. x?=w382:bool)
            }
          }
          frame #3 {
            w1169 = FALSE
            n406 = property on="Tab Control" class="TabCtl (strict)"("DisabledEnum"=T4."Enabled" ("Disabled")) -> ()  [unwired: 2 in, 2 out]
            n407 = call-poly <vilib>:"DAQmx Write.vi"("task/channels in"=w1172, "data"=FALSE) -> ()  [unwired: 11 in, 3 out]
            n408 = call-poly <vilib>:"DAQmx Write.vi"("task/channels in"=w1173, "data"=FALSE) -> ()  [unwired: 11 in, 3 out]
            n409 = VISA Write(VISA resource name=w1170, write buffer="la off\r" ("format string")) -> ()  [unwired: 1 in, 3 out]
            n410 = property on="561" class="Bool (strict)"("Value"=w1169) -> ()  [unwired: 2 in, 2 out]
            n411 = property on="488" class="Bool (strict)"("Value"=w1169) -> ()  [unwired: 2 in, 2 out]
            n412 = property on="405" class="Bool (strict)"("Value"=w1169) -> ()  [unwired: 2 in, 2 out]
            n413 = property on="647" class="Bool (strict)"("Value"=w1169) -> ()  [unwired: 2 in, 2 out]
          }
        }
      }
    }
    n414 = property on="stop" class="Bool (strict)"() -> ("Value"=w209:bool)  [unwired: 2 in, 2 out]
    n415 = Wait (ms)(milliseconds to wait=u32 100) -> ()  [unwired: 1 out]
  }
  n416 = VISA Write(VISA resource name=w33, write buffer="en 1\r" ("format string")) -> (VISA resource name out=w32:refnum<visa-resource-name>)  [unwired: 1 in, 2 out]
  n417 = property class="MG17Motor"(reference="MG17Motor", "HWSerialNum"=i64 83839541 ("Numeric 2")) -> (reference out=w40:refnum<k7>)  [unwired: 1 in, 1 out]
  n418 = invoke class="MG17Motor" method="StartCtrl"(reference=w40) -> (reference out=w39:refnum<k7>, error out=w38:errorcluster)  [unwired: 2 in, 1 out]
  n419 = while {
    tunnel: w75 -> [w1184]
    tunnel: w76 -> [w1185]
    tunnel: [w1185] -> w65
    tunnel: [w1184] -> w64
    tunnel: w32 -> [w1179]
    tunnel: w31 -> [w1182]
    tunnel: [w1181] -> w44
    tunnel: [w1180] -> w43
    tunnel: w6 -> [w1177]
    tunnel: [w1177] -> w5
    stop <- w1183 stop-if-true
    w1186 = 100
    n420 = Wait (ms)(milliseconds to wait=u32 250) -> ()  [unwired: 1 out]
    n421 = event shown="[0] Timeout" {
      selector: _ -> [_ _]
      dyn-events: _ -> [_ _]
      timeout: w1186 -> [_ _]
      tunnel: w1182 -> [_ w1233]
      event Timeout {
        n422 = event-data() -> ()  [unwired: 1 in, 3 out]
      }
      event "405": Value Change {
        n423 = event-data() -> ("NewVal"=w1234:bool)  [unwired: 1 in, 5 out]
        n424 = call-poly <vilib>:"DAQmx Write.vi"("task/channels in"=w1233, "data"=w1234) -> ()  [unwired: 11 in, 3 out]
      }
    }
    n425 = event shown="[2] \"488 power\": Mouse Up" {
      selector: _ -> [_ _ _]
      dyn-events: _ -> [_ _ _]
      timeout: w1186 -> [_ _ _]
      tunnel: w1184 -> [_ w1211 _]
      tunnel: w1177 -> [_ _ w1216]
      event Timeout {
        n426 = event-data() -> ()  [unwired: 1 in, 3 out]
      }
      event "488": Value Change {
        n427 = event-data() -> ("NewVal"=w1212:bool)  [unwired: 1 in, 5 out]
        n428 = call-poly <vilib>:"DAQmx Write.vi"("task/channels in"=w1211, "data"=w1212) -> ()  [unwired: 11 in, 3 out]
      }
      event "488 power": Mouse Up {
        n429 = event-data() -> ()  [unwired: 1 in, 1 out]
        n430 = Divide(x="488 power", y=200.0) -> (x/y=w1213:dbl)
        n431 = stacked-sequence {
          seq-local: [w1217 _ _ _] -> [_ _ w1229 _]
          seq-local: [_ _ w1228 _] -> [_ _ _ w1231]
          tunnel: w1213 -> [w1218 _ _ _]
          tunnel: w1216 -> [_ w1223 _ w1232]
          frame #0 {
            w1222 = "p"  # Command
            n432 = Number To Fractional String(use system decimal point (T)=FALSE, number=w1218) -> (F-format string=w1220:string)  [unwired: 2 in]
            n433 = call <vilib>:"Space Constant.vi"() -> ("String"=w1221:string)
            n434 = Concatenate Strings(w1222, w1221, w1220) -> (w1217:string)
          }
          frame #1 {
            n435 = VISA Flush I/O Buffer(VISA resource name=w1223, mask (16)=u16 128) -> (VISA resource name out=w1226:refnum<visa-resource-name>, error out=w1227:errorcluster)  [unwired: 1 in]
            n436 = VISA Flush I/O Buffer(VISA resource name=w1226, mask (16)=u16 64, error in (no error)=w1227) -> ()  [unwired: 2 out]
          }
          frame #2 {
            w1230 = "\r"  # StopChar
            n437 = Concatenate Strings(w1229, w1230) -> (w1228:string)
          }
          frame #3 {
            n438 = VISA Write(VISA resource name=w1232, write buffer=w1231) -> ()  [unwired: 1 in, 3 out]
          }
        }
      }
    }
    n439 = event shown="[1] \"561\": Value Change" {
      selector: _ -> [_ _]
      dyn-events: _ -> [_ _]
      timeout: w1186 -> [_ _]
      tunnel: w1185 -> [_ w1209]
      event Timeout {
        n440 = event-data() -> ()  [unwired: 1 in, 3 out]
      }
      event "561": Value Change {
        n441 = event-data() -> ("NewVal"=w1210:bool)  [unwired: 1 in, 5 out]
        n442 = call-poly <vilib>:"DAQmx Write.vi"("task/channels in"=w1209, "data"=w1210) -> ()  [unwired: 11 in, 3 out]
      }
    }
    n443 = event shown="[1] \"647\": Value Change" {
      selector: _ -> [_ _ _]
      dyn-events: _ -> [_ _ _]
      timeout: w1186 -> [_ _ _]
      tunnel: w1179 -> [w1187 w1190 w1204]
      tunnel: [_ w1189 w1201] -> w1180
      tunnel: [w1187 w1188 w1202] -> w1181
      event Timeout {
        n444 = event-data() -> ()  [unwired: 1 in, 3 out]
      }
      event "647": Value Change {
        n445 = event-data() -> ("NewVal"=w1191:bool)  [unwired: 1 in, 5 out]
        n446 = case shown="True" w1191 {
          tunnel: w1190 -> [w1193 w1198]
          tunnel: [w1194 w1197] -> w1189
          tunnel: [w1192 w1196] -> w1188
          frame False {
            n447 = VISA Write(VISA resource name=w1193, write buffer="la off\r" ("format string")) -> (VISA resource name out=w1192:refnum<visa-resource-name>, error out=w1194:errorcluster)  [unwired: 1 in, 1 out]
          }
          frame True {
            n448 = VISA Write(VISA resource name=w1198, write buffer="la on\r" ("format string")) -> (VISA resource name out=w1196:refnum<visa-resource-name>, error out=w1197:errorcluster)  [unwired: 1 in, 1 out]
          }
        }
      }
      event "647 Power": Mouse Up {
        n449 = event-data() -> ()  [unwired: 1 in, 1 out]
        n450 = To Unsigned Byte Integer(number="647 Power") -> (unsigned 8bit integer=w1208:u8)
        n451 = Number To Decimal String(number=w1208) -> (decimal integer string=w1206:string)  [unwired: 1 in]
        n452 = Concatenate Strings("ch 1 pow ", w1206, "\r") -> (w1203:string)
        n453 = VISA Write(VISA resource name=w1204, write buffer=w1203) -> (VISA resource name out=w1202:refnum<visa-resource-name>, error out=w1201:errorcluster)  [unwired: 1 in, 1 out]
      }
    }
    n454 = property on="stop" class="Bool (strict)"() -> ("Value"=w1183:bool)  [unwired: 2 in, 2 out]
  }
  n455 = while {
    tunnel: w8 -> [w1245]
    tunnel: w9 -> [w1244]
    tunnel: w3 -> [w1246]
    tunnel: ["stop"] -> _
    tunnel: [w1246] -> w73
    tunnel: [w1245] -> w72
    tunnel: [w1244] -> w74
    shift-right: [w1238] -> _
    shift-left: 0 -> [w1237]
    tunnel: w16 -> [w1235]
    tunnel: [w1235] -> w15
    stop <- "stop" stop-if-true
    n456 = Greater?(x=w1237, y=8) -> (0:w1240:bool)
    n457 = Select(t=0, s=w1240, f=w1237) -> (s? t:f=w1239:i32)
    n458 = Add(x=1, y=w1239) -> (x+y=w1238:i32)
    "x+y" <- w1238
    n459 = case shown="True" "Go live" {
      tunnel: w1246 -> [_ w1253]
      tunnel: w1245 -> [_ w1252]
      tunnel: w1244 -> [_ w1251]
      tunnel: w1238 -> [_ w1248]
      frame False {
      }
      frame True {
        n460 = property on="561 voltages" class="Arr (strict)"() -> ("Value"=w1249:dbl[][])  [unwired: 2 in, 2 out]
        n461 = case shown="\"Widefield\"" "Live mode" {
          tunnel: w1249 -> [_ _ w1364 w1402]
          tunnel: w1252 -> [_ w1292 w1350 w1396]
          tunnel: w1251 -> [w1255 w1295 w1352 _]
          tunnel: w1253 -> [w1254 w1296 w1351 _]
          tunnel: w1248 -> [_ _ w1340 _]
          frame "Static", Default {
            n462 = flat-sequence {
              tunnel: w1255 -> [w1268]
              tunnel: [w1266] -> w1263
              tunnel: [w1265] -> w1262
              tunnel: w1254 -> [w1264]
              tunnel: [w1264] -> w1261
              tunnel: w1263 -> [w1272]
              tunnel: [w1272] -> w1260
              tunnel: w1262 -> [w1270]
              tunnel: [w1271] -> w1259
              tunnel: w1261 -> [w1271]
              tunnel: [w1270] -> w1258
              tunnel: w1260 -> [w1277]
              tunnel: [w1275] -> w1257
              tunnel: w1259 -> [w1275]
              tunnel: w1258 -> [w1274]
              tunnel: [w1273] -> w1256
              tunnel: w1257 -> [w1280]
              tunnel: w1256 -> [w1279]
              tunnel: [w1278] -> _
              frame #0 {
                n463 = call-poly <vilib>:"DAQmx Write.vi"("task/channels in"=w1268, "data"=TRUE) -> ("task out"=w1266:refnum<k21>, "error out"=w1265:errorcluster)  [unwired: 11 in, 1 out]
              }
              frame #1 {
                n464 = property on="Exposure \n(ms)" class="DigNum (strict)"() -> ("Value"=w1269:dbl)  [unwired: 2 in, 2 out]
                n465 = Wait (ms)(milliseconds to wait=w1269) -> ()  [unwired: 1 out]
              }
              frame #2 {
                n466 = call-poly <vilib>:"DAQmx Write.vi"("task/channels in"=w1277, "data"=FALSE, "error in"=w1274) -> ("error out"=w1273:errorcluster)  [unwired: 10 in, 2 out]
              }
              frame #3 {
                n467 = while {
                  tunnel: w1280 -> [w1285]
                  tunnel: w1279 -> [w1284]
                  tunnel: [w1283] -> w1278
                  stop <- w1282 stop-if-true
                  n468 = call-poly <vilib>:"DAQmx Read.vi"("task/channels in"=w1285, "error in"=w1284) -> ("data"=w1281:bool, "error out"=w1283:errorcluster)  [unwired: 11 in, 1 out]
                  n469 = Not(x=w1281) -> (.not. x?=w1282:bool)
                }
              }
            }
          }
          frame "Widefield" {
            n470 = call <vilib>:"Sine Waveform.vi"("offset"=2.2, "sampling info"=cluster{"Fs":dbl, "#s":dbl} {"Fs"=10.0, "#s"=10.0}, "reset signal"=TRUE, "amplitude"=0.02, "frequency"=0.1) -> ("signal out"=w1286:waveform(dbl))  [unwired: 5 in, 1 out]
            n471 = call-poly <vilib>:"DAQmx Write.vi"("task/channels in"=w1292, "auto start"=TRUE, "data"=w1286) -> ("error out"=w1294:errorcluster)  [unwired: 10 in, 2 out]
            "error out" <- w1294
            n472 = while {
              tunnel: w1296 -> [w1305]
              tunnel: w1295 -> [w1304]
              tunnel: w1294 -> [w1297]
              stop <- w1303 stop-if-true
              n473 = flat-sequence {
                tunnel: w1304 -> [w1319]
                tunnel: [w1317] -> w1313
                tunnel: [w1316] -> w1312
                tunnel: [w1315] -> w1311
                tunnel: w1305 -> [w1315]
                tunnel: w1297 -> [w1314]
                tunnel: w1313 -> [w1323]
                tunnel: [w1323] -> w1310
                tunnel: w1312 -> [w1321]
                tunnel: [w1322] -> w1309
                tunnel: w1311 -> [w1322]
                tunnel: [w1321] -> w1308
                tunnel: w1310 -> [w1328]
                tunnel: [w1326] -> w1307
                tunnel: w1309 -> [w1326]
                tunnel: w1308 -> [w1325]
                tunnel: [w1324] -> w1306
                tunnel: w1307 -> [w1331]
                tunnel: w1306 -> [w1330]
                tunnel: [w1329] -> _
                frame #0 {
                  n474 = call-poly <vilib>:"DAQmx Write.vi"("task/channels in"=w1319, "data"=TRUE, "error in"=w1314) -> ("task out"=w1317:refnum<k21>, "error out"=w1316:errorcluster)  [unwired: 10 in, 1 out]
                }
                frame #1 {
                  n475 = property on="Exposure \n(ms)" class="DigNum (strict)"() -> ("Value"=w1320:dbl)  [unwired: 2 in, 2 out]
                  n476 = Wait (ms)(milliseconds to wait=w1320) -> ()  [unwired: 1 out]
                }
                frame #2 {
                  n477 = call-poly <vilib>:"DAQmx Write.vi"("task/channels in"=w1328, "data"=FALSE, "error in"=w1325) -> ("error out"=w1324:errorcluster)  [unwired: 10 in, 2 out]
                }
                frame #3 {
                  n478 = while {
                    tunnel: w1331 -> [w1336]
                    tunnel: w1330 -> [w1335]
                    tunnel: [w1334] -> w1329
                    stop <- w1333 stop-if-true
                    n479 = call-poly <vilib>:"DAQmx Read.vi"("task/channels in"=w1336, "error in"=w1335) -> ("data"=w1332:bool, "error out"=w1334:errorcluster)  [unwired: 11 in, 1 out]
                    n480 = Not(x=w1332) -> (.not. x?=w1333:bool)
                  }
                }
              }
              n481 = property on="Go live" class="Bool (strict)"() -> ("Value"=w1300:bool)  [unwired: 2 in, 2 out]
              n482 = property on="Live mode" class="RadioBtnsControl (strict)"() -> ("Value"=w1302:enum32{"Static", "Strobe", "Widefield", "SIM"})  [unwired: 2 in, 2 out]
              n483 = Equal?(x=w1302, y=enum32{"Static", "Strobe", "Widefield", "SIM"}."Widefield") -> (x = y?=w1299:bool)
              n484 = And(x=w1299, y=w1300) -> (x .and. y?=w1298:bool)
              n485 = Not(x=w1298) -> (.not. x?=w1303:bool)
            }
          }
          frame "SIM" {
            n486 = Quotient & Remainder(x=w1340, y=9) -> (x-y*floor(x/y)=w1362:i32)  [unwired: 1 out]
            n487 = flat-sequence {
              tunnel: w1351 -> [w1368]
              tunnel: w1352 -> [w1369]
              tunnel: [w1369] -> w1349
              tunnel: [w1365] -> w1347
              tunnel: [w1368] -> w1345
              tunnel: w1350 -> [w1367]
              tunnel: w1339 -> [w1366]
              tunnel: w1349 -> [w1373]
              tunnel: [w1373] -> w1348
              tunnel: w1347 -> [w1372]
              tunnel: [w1372] -> w1346
              tunnel: w1345 -> [w1371]
              tunnel: [w1371] -> w1344
              tunnel: [w1377] -> w1360
              tunnel: [w1375] -> w1359
              tunnel: [w1374] -> w1358
              tunnel: w1348 -> [w1379]
              tunnel: w1346 -> [w1376]
              tunnel: w1344 -> [w1374]
              tunnel: w1360 -> [w1383]
              tunnel: [w1383] -> w1357
              tunnel: w1359 -> [w1381]
              tunnel: [w1382] -> w1356
              tunnel: w1358 -> [w1382]
              tunnel: [w1381] -> w1355
              tunnel: w1357 -> [w1388]
              tunnel: [w1386] -> w1354
              tunnel: w1356 -> [w1386]
              tunnel: w1355 -> [w1385]
              tunnel: [w1384] -> w1353
              tunnel: w1354 -> [w1390]
              tunnel: w1353 -> [w1389]
              frame #0 {
                n488 = call-poly <vilib>:"DAQmx Write.vi"("task/channels in"=w1367, "data"=w1366) -> ("error out"=w1365:errorcluster)  [unwired: 11 in, 2 out]
              }
              frame #1 {
                n489 = property on="Delay time" class="DigNum (strict)"() -> ("Value"=w1370:u32)  [unwired: 2 in, 2 out]
                n490 = Wait (ms)(milliseconds to wait=w1370) -> ()  [unwired: 1 out]
              }
              frame #2 {
                n491 = call-poly <vilib>:"DAQmx Write.vi"("task/channels in"=w1379, "data"=TRUE, "error in"=w1376) -> ("task out"=w1377:refnum<k21>, "error out"=w1375:errorcluster)  [unwired: 10 in, 1 out]
              }
              frame #3 {
                n492 = property on="Exposure \n(ms)" class="DigNum (strict)"() -> ("Value"=w1380:dbl)  [unwired: 2 in, 2 out]
                n493 = Wait (ms)(milliseconds to wait=w1380) -> ()  [unwired: 1 out]
              }
              frame #4 {
                n494 = call-poly <vilib>:"DAQmx Write.vi"("task/channels in"=w1388, "data"=FALSE, "error in"=w1385) -> ("error out"=w1384:errorcluster)  [unwired: 10 in, 2 out]
              }
              frame #5 {
                n495 = while {
                  tunnel: w1390 -> [w1395]
                  tunnel: w1389 -> [w1394]
                  tunnel: [w1393] -> _
                  stop <- w1392 stop-if-true
                  n496 = call-poly <vilib>:"DAQmx Read.vi"("task/channels in"=w1395, "error in"=w1394) -> ("data"=w1391:bool, "error out"=w1393:errorcluster)  [unwired: 11 in, 1 out]
                  n497 = Not(x=w1391) -> (.not. x?=w1392:bool)
                }
              }
            }
            n498 = Add(x=0, y=w1362) -> (x+y=w1341:i32)
            n499 = Index Array(array=i32[] [1, 2, 0, 1, 2, 0, 1, 2, 0, 0, 1, 2, 3, 4, 0], index=w1341) -> (element=w1337:i32)
            n500 = Index Array(array=i32[] [0, 0, 1, 1, 1, 2, 2, 2, 0, 2, 2, 2, 2, 2, 0], index=w1341) -> (element=w1338:i32)
            n501 = Index Array(array=w1364, index (row)=w1337, index (col)=w1338) -> (element=w1339:dbl)
            n502 = property on="Current voltage" class="DigNum (strict)"("Value"=w1339) -> ()  [unwired: 2 in, 2 out]
          }
          frame "Strobe" {
            n503 = flat-sequence {
              tunnel: w1402 -> [w1404]
              tunnel: [w1404] -> w1400
              tunnel: w1396 -> [w1403]
              tunnel: [w1409] -> w1401
              tunnel: w1400 -> [w1409]
              tunnel: w1401 -> [w1411]
              tunnel: [w1411] -> w1399
              tunnel: w1396 -> [w1410]
              tunnel: w1399 -> [w1416]
              tunnel: [w1416] -> w1398
              tunnel: w1398 -> [w1418]
              tunnel: [w1418] -> w1397
              tunnel: w1396 -> [w1417]
              tunnel: [w1423] -> _
              tunnel: w1397 -> [w1423]
              frame #0 {
                n504 = Index Array(array=w1404, index (row)=2, index (col)=0) -> (element=w1405:dbl)
                n505 = call-poly <vilib>:"DAQmx Write.vi"("task/channels in"=w1403, "data"=w1405) -> ()  [unwired: 11 in, 3 out]
              }
              frame #1 {
                n506 = property on="Delay time" class="DigNum (strict)"() -> ("Value"=w1408:u32)  [unwired: 2 in, 2 out]
                n507 = Wait (ms)(milliseconds to wait=w1408) -> ()  [unwired: 1 out]
              }
              frame #2 {
                n508 = Index Array(array=w1411, index (row)=2, index (col)=1) -> (element=w1414:dbl)
                n509 = call-poly <vilib>:"DAQmx Write.vi"("task/channels in"=w1410, "data"=w1414) -> ()  [unwired: 11 in, 3 out]
              }
              frame #3 {
                n510 = property on="Delay time" class="DigNum (strict)"() -> ("Value"=w1415:u32)  [unwired: 2 in, 2 out]
                n511 = Wait (ms)(milliseconds to wait=w1415) -> ()  [unwired: 1 out]
              }
              frame #4 {
                n512 = Index Array(array=w1418, index (row)=2, index (col)=2) -> (element=w1419:dbl)
                n513 = call-poly <vilib>:"DAQmx Write.vi"("task/channels in"=w1417, "data"=w1419) -> ()  [unwired: 11 in, 3 out]
              }
              frame #5 {
                n514 = property on="Delay time" class="DigNum (strict)"() -> ("Value"=w1422:u32)  [unwired: 2 in, 2 out]
                n515 = Wait (ms)(milliseconds to wait=w1422) -> ()  [unwired: 1 out]
              }
            }
          }
        }
      }
    }
    "?" <- "Go live"
  }
  n516 = stacked-sequence {
    tunnel: w39 -> [w1426 w1444]
    tunnel: w38 -> [w1425 _]
    tunnel: [_ w1443] -> w37
    tunnel: [_ w1442] -> _
    frame #0 {
      n517 = invoke class="MG17Motor" method="SetVelParams"(reference=w1426, error in=w1425, "lChanID"=0, "fMinVel"=0.0, "fAccn"=20, "fMaxVel"=20) -> (reference out=w1433:refnum<k7>, error out=w1432:errorcluster)  [unwired: 1 in, 5 out]
      n518 = property on="561 power" class="Slide (strict)"() -> ("Value"=w1428:dbl)  [unwired: 2 in, 2 out]
      n519 = Multiply(x=45, y=w1428) -> (x*y=w1429:dbl)
      n520 = Add(x=78, y=w1429) -> (x+y=w1427:dbl)
      n521 = invoke class="MG17Motor" method="SetAbsMovePos"(reference=w1433, error in=w1432, "lChanID"=0, "fAbsPos"=w1427) -> (reference out=w1435:refnum<k7>, error out=w1434:errorcluster)  [unwired: 1 in, 3 out]
      n522 = invoke class="MG17Motor" method="MoveAbsolute"(reference=w1435, error in=w1434, "lChanID"=0, "bWait"=TRUE) -> ()  [unwired: 1 in, 5 out]
    }
    frame #1 {
      n523 = while {
        tunnel: [w1453] -> w1443
        tunnel: w1444 -> [w1451]
        tunnel: [w1450] -> w1442
        stop <- w1449 stop-if-true
        n524 = Wait (ms)(milliseconds to wait=250) -> ()  [unwired: 1 out]
        n525 = Divide(x="561 power", y=100.0) -> (x/y=w1445:dbl)
        n526 = event shown="[0] Timeout" {
          selector: _ -> [_ _]
          dyn-events: _ -> [_ _]
          timeout: 10 -> [_ _]
          tunnel: w1451 -> [w1454 w1462]
          tunnel: [w1454 w1461] -> w1453
          tunnel: w1445 -> [_ w1457]
          tunnel: [_ w1464] -> w1450
          event Timeout {
            n527 = event-data() -> ()  [unwired: 1 in, 3 out]
          }
          event "561 power": Mouse Up {
            n528 = event-data() -> ()  [unwired: 1 in, 4 out]
            n529 = Multiply(x=45, y=w1457) -> (x*y=w1458:dbl)
            n530 = Add(x=81 ("561 power offset"), y=w1458) -> (x+y=w1456:dbl)
            n531 = invoke class="MG17Motor" method="SetAbsMovePos"(reference=w1462, "lChanID"=0, "fAbsPos"=w1456) -> (reference out=w1460:refnum<k7>)  [unwired: 2 in, 4 out]
            n532 = invoke class="MG17Motor" method="MoveAbsolute"(reference=w1460, "lChanID"=0, "bWait"=TRUE) -> (reference out=w1461:refnum<k7>, error out=w1464:errorcluster)  [unwired: 2 in, 3 out]
          }
        }
        n533 = property on="stop" class="Bool (strict)"() -> ("Value"=w1449:bool)  [unwired: 2 in, 2 out]
      }
    }
  }
  n534 = invoke class="MG17Motor" method="StopCtrl"(reference=w37) -> ()  [unwired: 2 in, 3 out]
  n535 = VISA Close(VISA resource name=w5) -> (error out=w4:errorcluster)  [unwired: 1 in]
  n536 = call <vilib>:"DAQmx Stop Task.vi"("task/channels in"=w15) -> ("task out"=w14:refnum<k21>)  [unwired: 13 in, 1 out]
  n537 = VISA Close(VISA resource name=w44, error in (no error)=w43) -> (error out=w42:errorcluster)
  n538 = call <vilib>:"DAQmx Clear Task.vi"("task in"=w14) -> ("error out"=w13:errorcluster)  [unwired: 14 in]
  n539 = call <vilib>:"DAQmx Stop Task.vi"("task/channels in"=w74) -> ("task out"=w69:refnum<k21>)  [unwired: 13 in, 1 out]
  n540 = call <vilib>:"DAQmx Stop Task.vi"("task/channels in"=w72) -> ("task out"=w71:refnum<k21>)  [unwired: 13 in, 1 out]
  n541 = call-poly <vilib>:"DAQmx Write.vi"("task/channels in"=w64, "data"=w63) -> ("task out"=w60:refnum<k21>, "error out"=w58:errorcluster)  [unwired: 11 in, 1 out]
  n542 = call-poly <vilib>:"DAQmx Write.vi"("task/channels in"=w65, "data"=w63) -> ("task out"=w59:refnum<k21>, "error out"=w57:errorcluster)  [unwired: 11 in, 1 out]
  n543 = call <vilib>:"DAQmx Stop Task.vi"("task/channels in"=w73) -> ("task out"=w70:refnum<k21>)  [unwired: 13 in, 1 out]
  n544 = call <vilib>:"DAQmx Clear Task.vi"("task in"=w69) -> ("error out"=w27:errorcluster)  [unwired: 14 in]
  n545 = call <vilib>:"DAQmx Clear Task.vi"("task in"=w71) -> ("error out"=w67:errorcluster)  [unwired: 14 in]
  n546 = property on="Go live" class="Bool (strict)"(error in=w27, "Value"=FALSE) -> (error out=w26:errorcluster)  [unwired: 1 in, 1 out]
  n547 = call <vilib>:"DAQmx Clear Task.vi"("task in"=w70) -> ("error out"=w66:errorcluster)  [unwired: 14 in]
  n548 = call <vilib>:"DAQmx Stop Task.vi"("task/channels in"=w60, "error in"=w58) -> ("task out"=w61:refnum<k21>, "error out"=w55:errorcluster)  [unwired: 12 in]
  n549 = call <vilib>:"DAQmx Stop Task.vi"("task/channels in"=w59, "error in"=w57) -> ("task out"=w62:refnum<k21>, "error out"=w56:errorcluster)  [unwired: 12 in]
  n550 = Merge Errors(w67, w66, w26, w13) -> (→"Camera/galvo error":errorcluster)
  n551 = call <vilib>:"DAQmx Clear Task.vi"("task in"=w62, "error in"=w56) -> ("error out"=w53:errorcluster)  [unwired: 13 in]
  n552 = call <vilib>:"DAQmx Clear Task.vi"("task in"=w61, "error in"=w55) -> ("error out"=w54:errorcluster)  [unwired: 13 in]
  n553 = Merge Errors(w53, w54, w42, w4) -> (→"Laser error":errorcluster)
  n554 = VISA Close(VISA resource name=w50) -> ()  [unwired: 1 in, 1 out]
